vi "ALONE_3AXIS_AMI_DESIM.vi"(6 "Refresco(s)":dbl=1.0, 8 "error in (no error)":errorcluster) -> (0 "Error Out":errorcluster, 7 "Enable":bool=TRUE)   [LabVIEW 2017]
uses:
  AMI MAGNET/Status AMI.ctl
  AMI MAGNET/magneticField.ctl
  ALONE_3AXIS_AMI.ctl
  AMI MAGNET/AMI 430_Hardware_Module.ctl
  AMI MAGNET/commsControl.ctl
  cRIO_ZNB_AMI_GLOBALES.vi
panel:
  in  "Demag X":bool
  out "Remote DEMAG Z":bool
  out "Remote DEMAG X":bool
  out "Remote DEMAG Y":bool
  in  "Demag Y":bool
  in  "Demag Z":bool
  out "String":string="Estado"
  out "Command":T1
  out "Remote RAMP Z":bool
  out "Remote SET X":bool
  out "Remote SET Y":bool
  out "Remote RAMP X":bool
  out "Remote RAMP Y":bool
  out "Remote SET Z":bool
  in  "rampingMode X":u16(ring)=1 items=["RAMP", "PAUSE", "MANUAL UP", "MANUAL DOWN", "ZERO"]
  in  "rampingMode Y":u16(ring)=1 items=["RAMP", "PAUSE", "MANUAL UP", "MANUAL DOWN", "ZERO"]
  in  "rampingMode Z":u16(ring)=1 items=["RAMP", "PAUSE", "MANUAL UP", "MANUAL DOWN", "ZERO"]
  in  "RAMP Z":bool
  in  "SET X":bool
  out "X ramping":bool caption="Stable"
  out "X state":T2=1 items=["Unknown", "RAMPING to target field/current", "HOLDING at the target field/current", "PAUSED", "Ramping in MANUAL UP mode", "Ramping in MANUAL DOWN mode", "ZEROING CURRENT (in progress)", "Quench detected", "At ZERO current", "Heating persistent switch", "Cooling persistent switch", "External Rampdown active"]
  in  "Target X(T)":dbl min=-0.5 max=0.5 step=0.001 format="%.3f"
  in  "Rate X(T/min)":dbl=0.1 min=0.0 max=0.1 step=0.001 format="%.3f"
  out "X field (T)":dbl format="%.3f"
  in  "SET Y":bool
  out "Y ramping":bool caption="Stable"
  out "Y state":T2=1 items=["Unknown", "RAMPING to target field/current", "HOLDING at the target field/current", "PAUSED", "Ramping in MANUAL UP mode", "Ramping in MANUAL DOWN mode", "ZEROING CURRENT (in progress)", "Quench detected", "At ZERO current", "Heating persistent switch", "Cooling persistent switch", "External Rampdown active"]
  in  "Target Y(T)":dbl min=-0.5 max=0.5 step=0.001 format="%.3f"
  in  "Rate Y(T/min)":dbl=0.1 min=0.0 max=0.1 step=0.001 format="%.3f"
  out "Y field (T)":dbl format="%.3f"
  in  "RAMP X":bool
  in  "RAMP Y":bool
  in  "Settings Z":T3={"magneticFieldUnits"=1, "rampRateUnits"=1, "rampRate"=0.0, "targetField"=0.0, "rampingMode"=1} {"rampingMode" items=["RAMP", "PAUSE", "MANUAL UP", "MANUAL DOWN", "ZERO"]; "targetField" format="%.3f"; "rampRate" format="%.3f"; "rampRateUnits" items=["Per SECOND", "Per MINUTE"]; "magneticFieldUnits" items=["KGauss", "Tesla"]}
  in  "Settings Y":T3={"magneticFieldUnits"=1, "rampRateUnits"=1, "rampRate"=0.0, "targetField"=0.0, "rampingMode"=1} {"rampingMode" items=["RAMP", "PAUSE", "MANUAL UP", "MANUAL DOWN", "ZERO"]; "targetField" format="%.3f"; "rampRate" format="%.3f"; "rampRateUnits" items=["Per SECOND", "Per MINUTE"]; "magneticFieldUnits" items=["KGauss", "Tesla"]}
  in  "Settings X":T3={"magneticFieldUnits"=1, "rampRateUnits"=1, "rampRate"=0.0, "targetField"=0.0, "rampingMode"=1} {"rampingMode" items=["RAMP", "PAUSE", "MANUAL UP", "MANUAL DOWN", "ZERO"]; "targetField" format="%.3f"; "rampRate" format="%.3f"; "rampRateUnits" items=["Per SECOND", "Per MINUTE"]; "magneticFieldUnits" items=["KGauss", "Tesla"]}
  out "Waveform Chart":T4(graph)
  in  "SET Z":bool
  out "Z ramping":bool caption="Stable"
  out "Z state":T2=1 items=["Unknown", "RAMPING to target field/current", "HOLDING at the target field/current", "PAUSED", "Ramping in MANUAL UP mode", "Ramping in MANUAL DOWN mode", "ZEROING CURRENT (in progress)", "Quench detected", "At ZERO current", "Heating persistent switch", "Cooling persistent switch", "External Rampdown active"]
  out "Ciclo":i32
  in  "Target Z(T)":dbl min=-2.0 max=2.0 step=0.001 format="%.3f"
  in  "Rate Z(T/min)":dbl=0.1 min=0.0 max=0.1 step=0.001 format="%.3f"
  out "Z field (T)":dbl format="%.3f"
  out "ERROR":bool
  out "Date":string caption="asd"
  out "Time":string caption="asd"
  in  "Refresh":bool
  in  "stop":bool
  # "Z axis"
  # "Y axis"
  # "X axis"
  # "STATUS"
  # "STATUS"
  # "STATUS"
  # "SETTINGS"
  # "SETTINGS"
  # "SETTINGS"
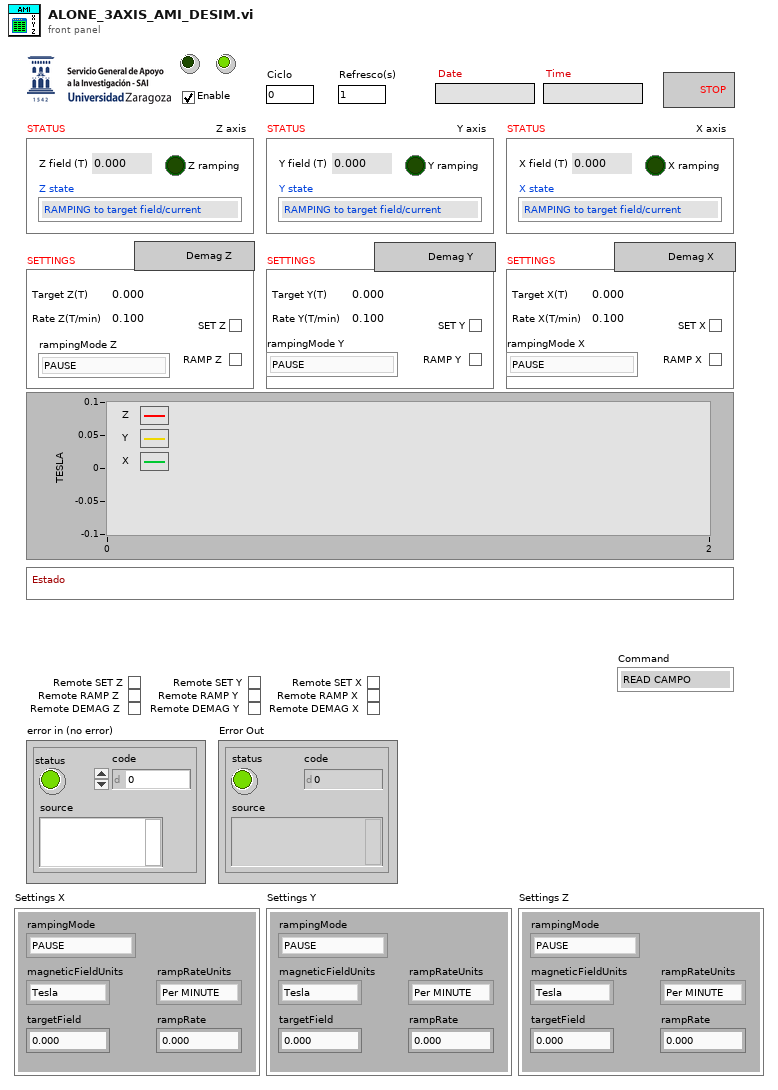
[diagram p1: front panel]
types:
  T1 = typedef "ALONE_3AXIS_AMI.ctl" = enum16{"READ CAMPO", "SET X", "SET Y", "SET Z", "RAMP X", "RAMP Y", "RAMP Z", "DESIMANAR X", "DESIMANAR Y", "DESIMANAR Z", "DESIMANAR X_RUN", "DESIMANAR Y_RUN", "DESIMANAR Z_RUN"}
  T2 = typedef "Status AMI.ctl" = u16
  T3 = typedef "magneticField.ctl" = cluster{"magneticFieldUnits":u16, "rampRateUnits":u16, "rampRate":dbl, "targetField":dbl, "rampingMode":u16}
  T4 = cluster{"magneticField":dbl, "magneticField":dbl, "magneticField":dbl}
  T5 = typedef "AMI 430_Hardware_Module.ctl" = enum16{"INICIALIZAR", "SET UNIDADES CAMPO", "SET UNIDADES RAMPA", "SET CAMPO", "SET  RAMPA", "SET RAMPING MODE", "READ CAMPO", "STATUS", "SHUTDOWN"}
  T6 = typedef "commsControl.ctl" = cluster{"connection ID":refnum<k5>, "IP":string, "Active Comm Interface":u16, "Serial Port":refnum<visa-resource-name>, "Programmer Type":u16, "connection ID":refnum<k5>, "output cluster":cluster{"GPIB address":i16, "GPIB bus":i16}}
  T7 = cluster{"Z field (T)":dbl, "Y field (T)":dbl, "magneticField":dbl}
  T8 = cluster{"Z field (T)":dbl, "magneticField":dbl, "X field (T)":dbl}
  T9 = cluster{"magneticField":dbl, "Y field (T)":dbl, "X field (T)":dbl}
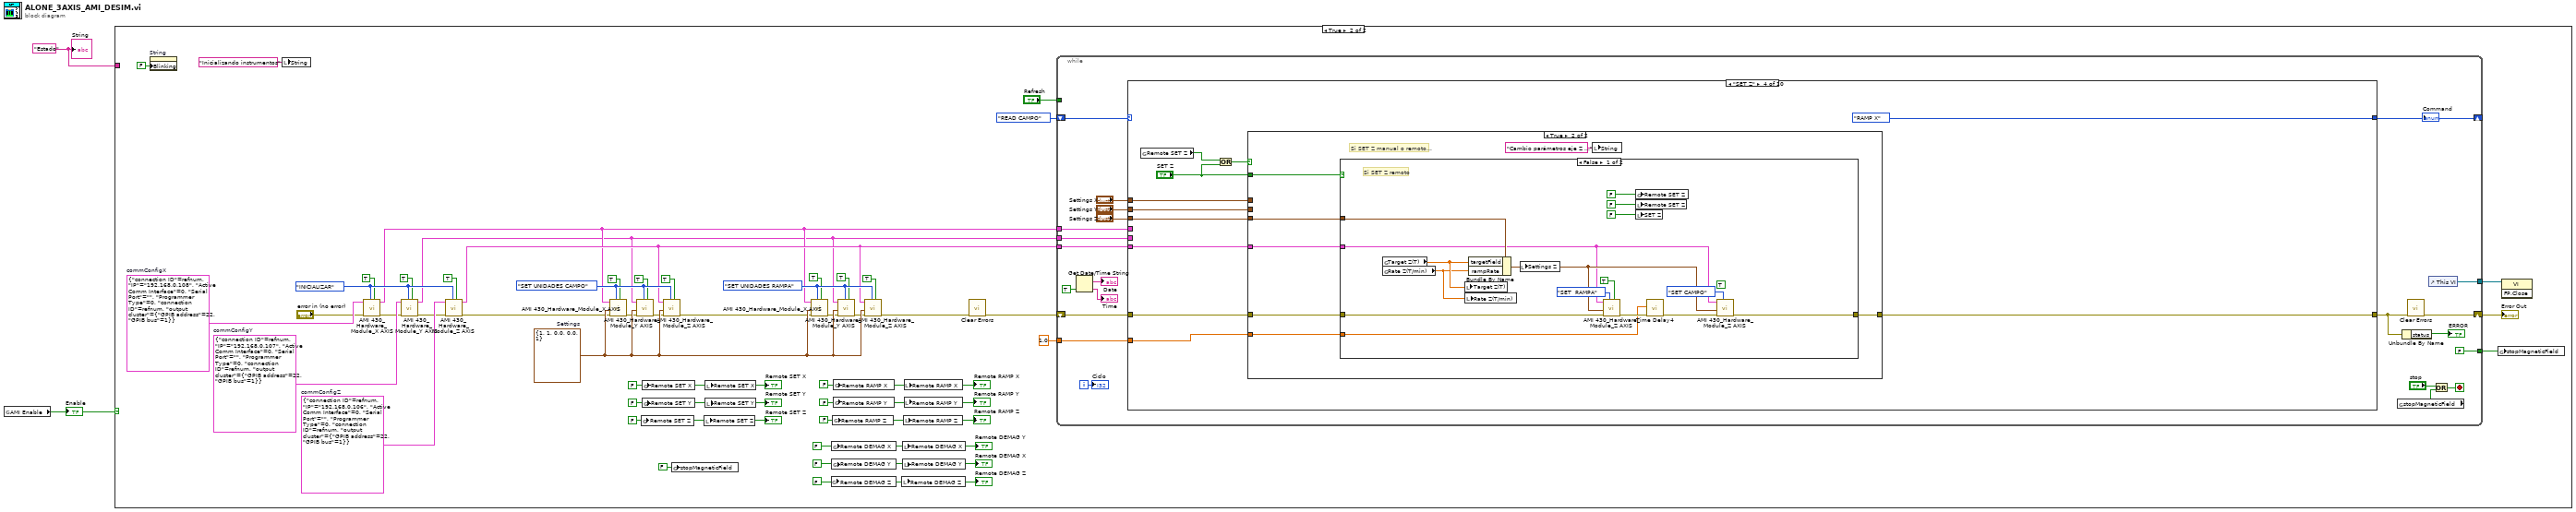
[diagram p0: block diagram]
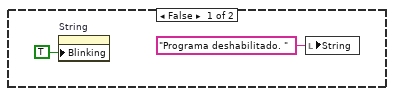
[diagram p2: hidden frame]
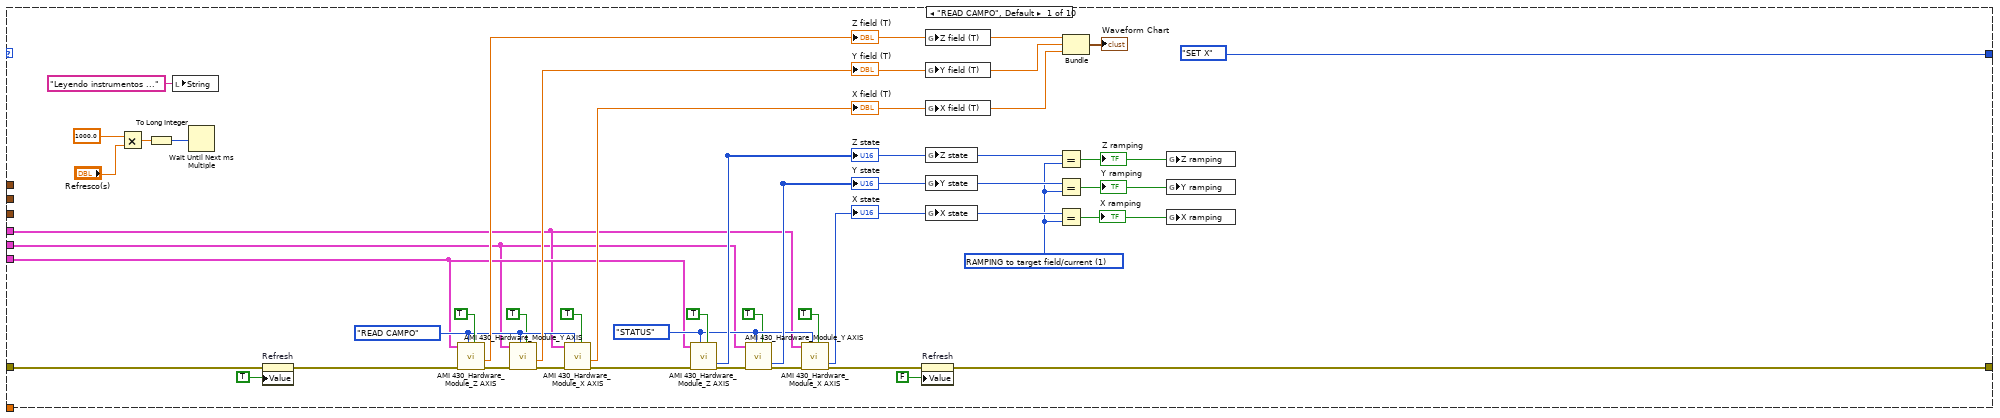
[diagram p3: hidden frame]
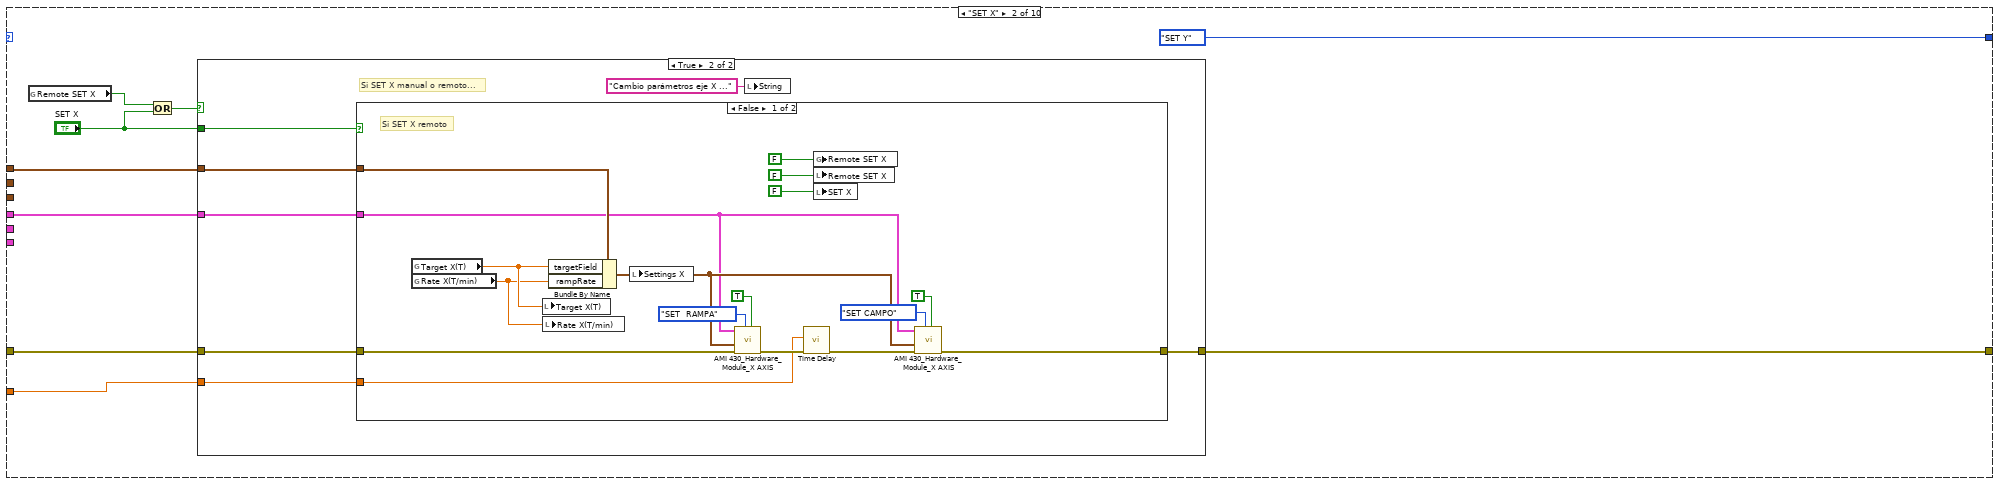
[diagram p4: hidden frame]
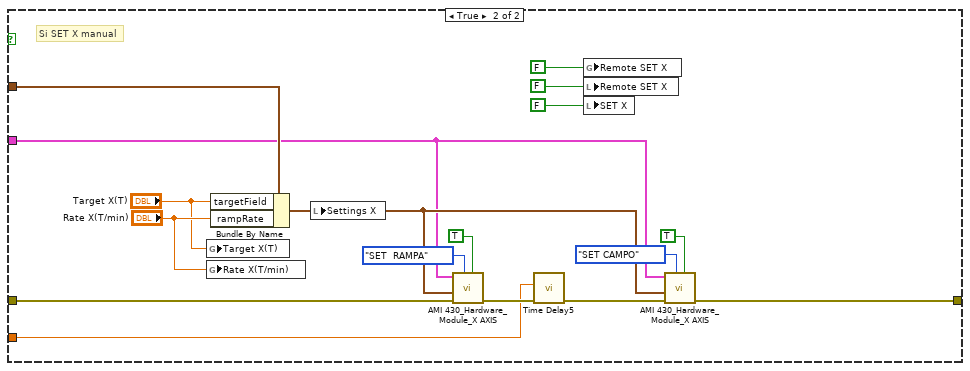
[diagram p6: hidden frame]
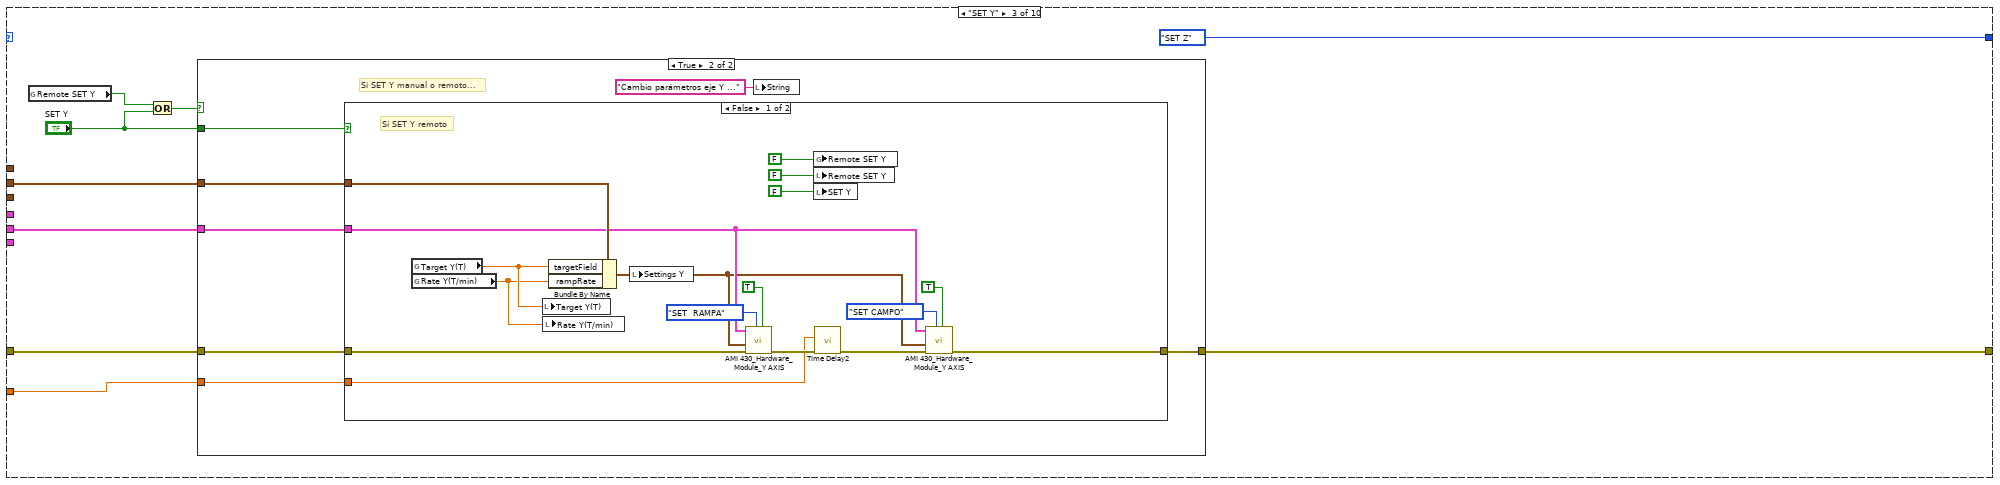
[diagram p7: hidden frame]
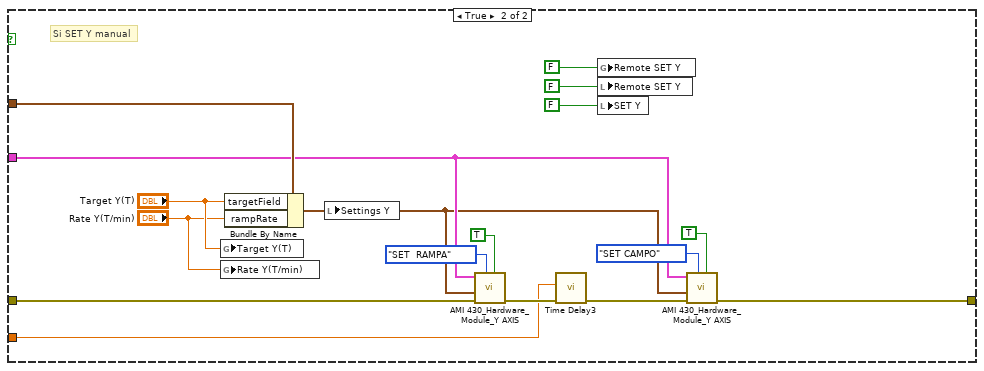
[diagram p9: hidden frame]
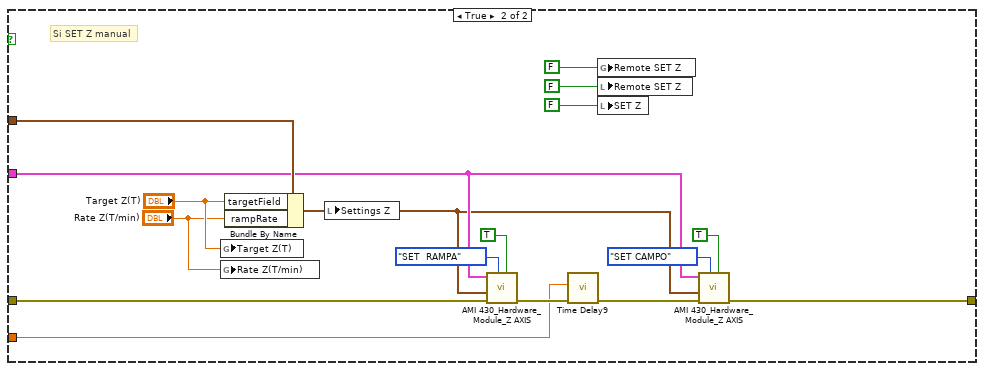
[diagram p11: hidden frame]
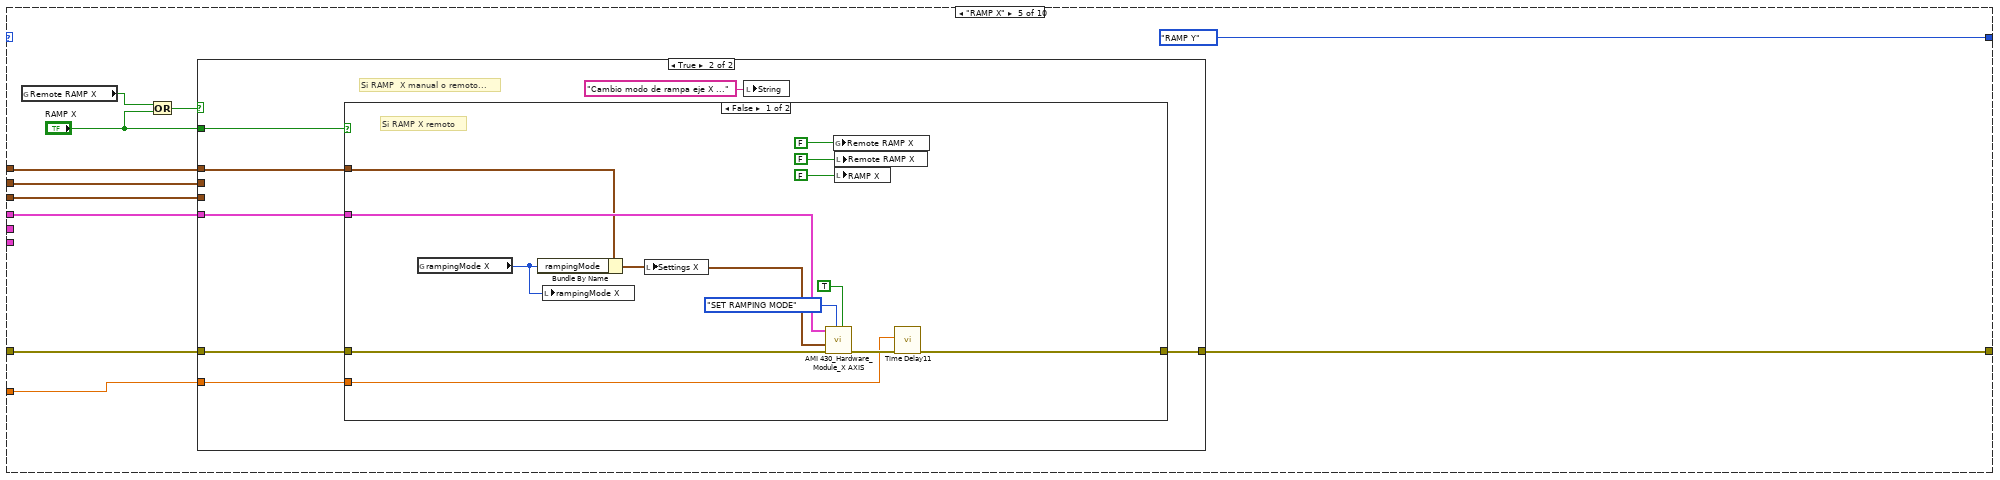
[diagram p12: hidden frame]
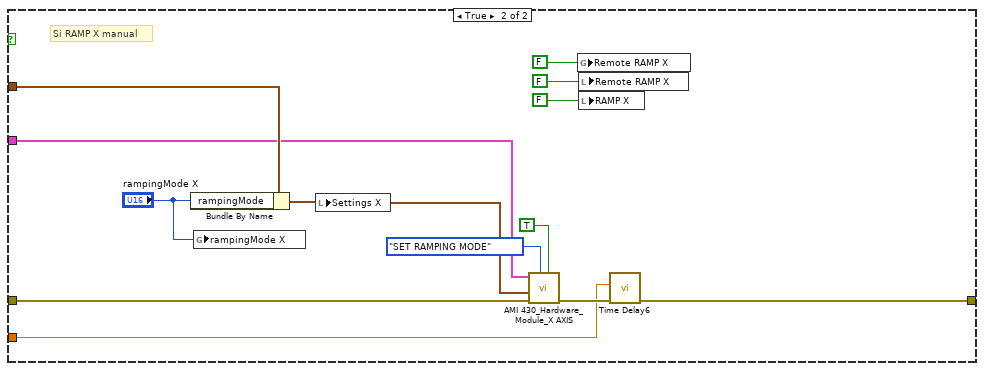
[diagram p14: hidden frame]
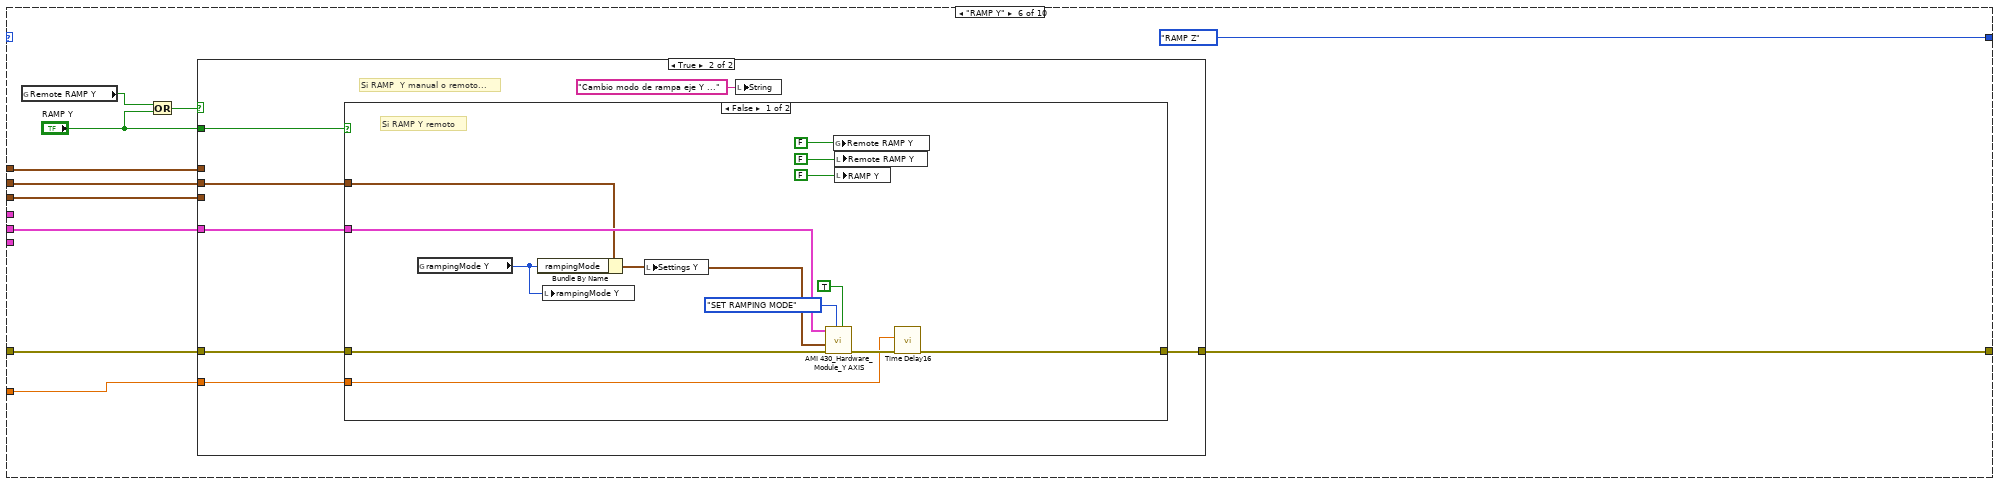
[diagram p15: hidden frame]
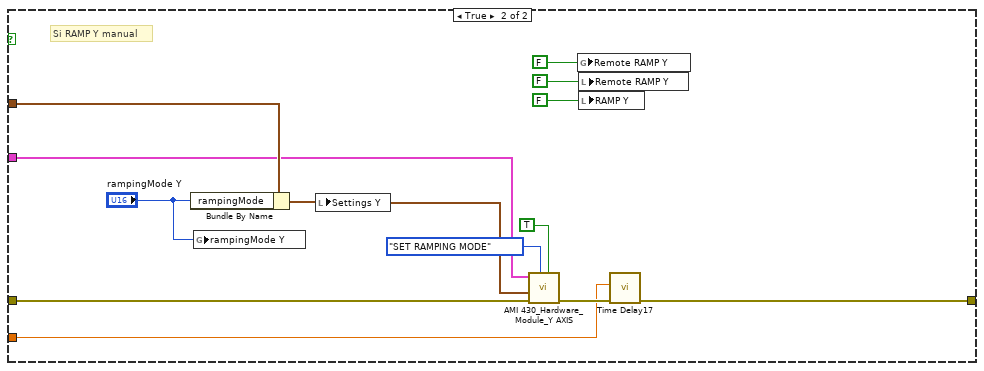
[diagram p17: hidden frame]
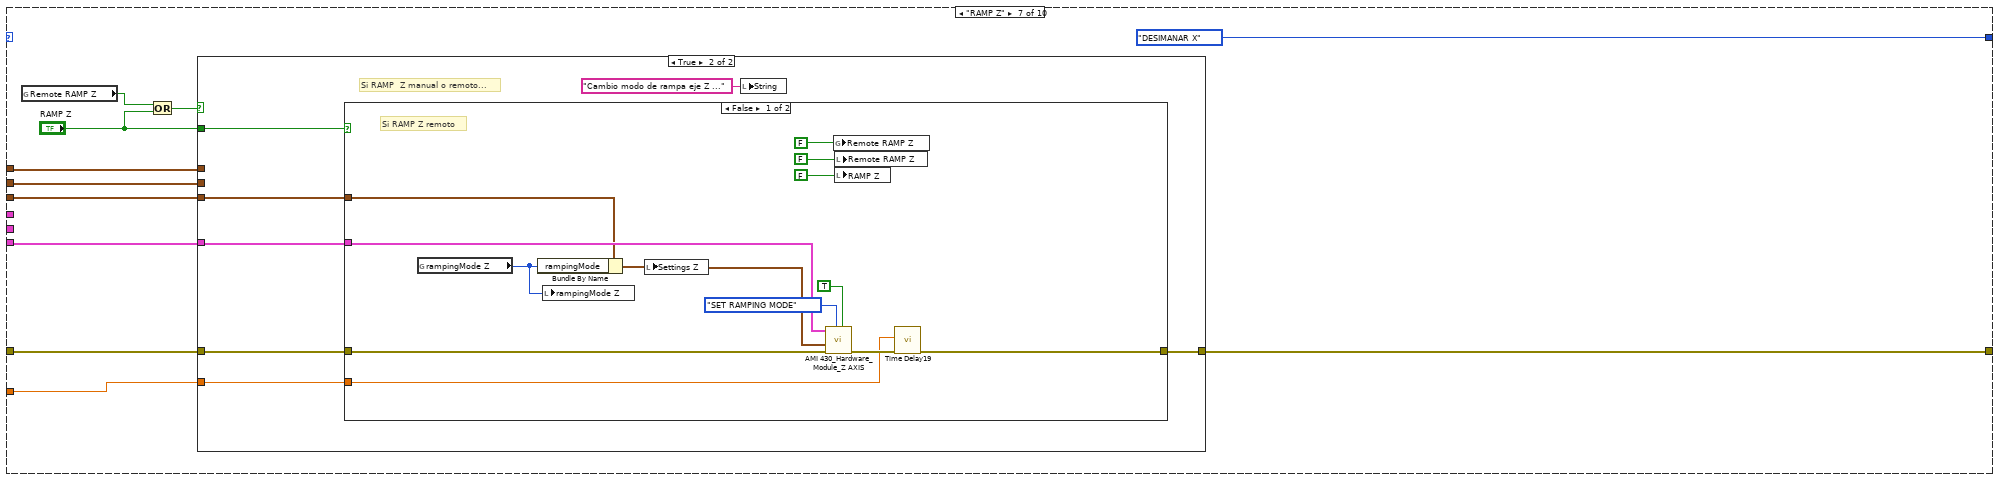
[diagram p18: hidden frame]
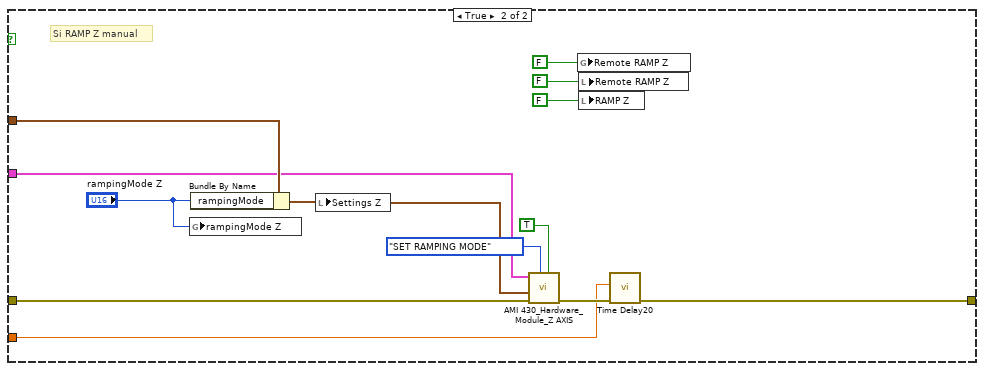
[diagram p20: hidden frame]
diagram:
  w1 = "Estado" ("String")
  n1 = global read "cRIO_ZNB_AMI_GLOBALES.vi" "AMI Enable"() -> (w2:bool)
  "Enable" <- w2
  n2 = case shown="True" w2 {
    tunnel: w1 -> [_ _]
    frame False {
      n3 = property on="String" class="Str"("Blinking"=TRUE) -> ()  [unwired: 2 in, 2 out]
      n4 = local write "String"("Programa deshabilitado. " ("String")) -> ()
    }
    frame True {
      w5 = FALSE ("Remote RAMP Z")
      w6 = FALSE ("Remote RAMP Y")
      w7 = FALSE ("Remote RAMP X")
      w12 = FALSE ("Remote SET Z")
      w11 = FALSE ("Remote SET Y")
      w13 = FALSE ("Remote SET X")
      w16 = FALSE ("Remote RAMP Z")
      w15 = FALSE ("Remote RAMP Y")
      w14 = FALSE ("Remote RAMP X")
      w45 = T3 {"magneticFieldUnits"=1, "rampRateUnits"=1, "rampRate"=0.0, "targetField"=0.0, "rampingMode"=1}  # Settings
      w41 = AMI_430_Hardware_Module."SET UNIDADES RAMPA" ("Command")
      w40 = AMI_430_Hardware_Module."SET UNIDADES CAMPO" ("Command")
      w48 = T6 {"connection ID"=refnum, "IP"="192.168.0.106", "Active Comm Interface"=0, "Serial Port"="", "Programmer Type"=0, "connection ID"=refnum, "output cluster"={"GPIB address"=22, "GPIB bus"=1}}  # commConfigZ
      w47 = T6 {"connection ID"=refnum, "IP"="192.168.0.107", "Active Comm Interface"=0, "Serial Port"="", "Programmer Type"=0, "connection ID"=refnum, "output cluster"={"GPIB address"=22, "GPIB bus"=1}}  # commConfigY
      w46 = T6 {"connection ID"=refnum, "IP"="192.168.0.108", "Active Comm Interface"=0, "Serial Port"="", "Programmer Type"=0, "connection ID"=refnum, "output cluster"={"GPIB address"=22, "GPIB bus"=1}}  # commConfigX
      w49 = AMI_430_Hardware_Module."INICIALIZAR" ("Command")
      n5 = property on="String" class="Str"("Blinking"=FALSE) -> ()  [unwired: 2 in, 2 out]
      n6 = local write "String"("Inicializando instrumentos" ("String")) -> ()
      n7 = call "AMI 430_Hardware_Module_X AXIS.vi"("Enable"=TRUE, "Command"=w49, "error in (no error)"="error in (no error)", "Comm Config In"=w46) -> ("error out"=w36:errorcluster, "Comm Config Out"=w20:T6)  [unwired: 3 in, 3 out]
      n8 = call "AMI 430_Hardware_Module_Y AXIS.vi"("Enable"=TRUE, "Command"=w49, "error in (no error)"=w36, "Comm Config In"=w47) -> ("error out"=w35:errorcluster, "Comm Config Out"=w19:T6)  [unwired: 3 in, 3 out]
      n9 = call "AMI 430_Hardware_Module_Z AXIS.vi"("Enable"=TRUE, "Command"=w49, "error in (no error)"=w35, "Comm Config In"=w48) -> ("error out"=w39:errorcluster, "Comm Config Out"=w21:T6)  [unwired: 3 in, 3 out]
      n10 = call "AMI 430_Hardware_Module_X AXIS.vi"("Enable"=TRUE, "Command"=w40, "error in (no error)"=w39, "Settings"=w45, "Comm Config In"=w20) -> ("error out"=w37:errorcluster)  [unwired: 2 in, 4 out]
      n11 = call "AMI 430_Hardware_Module_Y AXIS.vi"("Enable"=TRUE, "Command"=w40, "error in (no error)"=w37, "Settings"=w45, "Comm Config In"=w19) -> ("error out"=w38:errorcluster)  [unwired: 2 in, 4 out]
      n12 = global write "cRIO_ZNB_AMI_GLOBALES.vi" "Remote SET Z"(w12) -> ()
      n13 = global write "cRIO_ZNB_AMI_GLOBALES.vi" "Remote SET X"(w13) -> ()
      n14 = global write "cRIO_ZNB_AMI_GLOBALES.vi" "Remote SET Y"(w11) -> ()
      n15 = call "AMI 430_Hardware_Module_Z AXIS.vi"("Enable"=TRUE, "Command"=w40, "error in (no error)"=w38, "Settings"=w45, "Comm Config In"=w21) -> ("error out"=w44:errorcluster)  [unwired: 2 in, 4 out]
      n16 = global write "cRIO_ZNB_AMI_GLOBALES.vi" "stopMagneticField"(FALSE ("stopMagneticField")) -> ()
      n17 = local write "Remote SET Z"(w12) -> ()
      n18 = local write "Remote SET X"(w13) -> ()
      n19 = local write "Remote SET Y"(w11) -> ()
      n20 = call "AMI 430_Hardware_Module_X AXIS.vi"("Enable"=TRUE, "Command"=w41, "error in (no error)"=w44, "Settings"=w45, "Comm Config In"=w20) -> ("error out"=w42:errorcluster)  [unwired: 2 in, 4 out]
      n21 = global write "cRIO_ZNB_AMI_GLOBALES.vi" "Remote DEMAG Z"(w5) -> ()
      n22 = global write "cRIO_ZNB_AMI_GLOBALES.vi" "Remote DEMAG X"(w7) -> ()
      n23 = global write "cRIO_ZNB_AMI_GLOBALES.vi" "Remote DEMAG Y"(w6) -> ()
      n24 = global write "cRIO_ZNB_AMI_GLOBALES.vi" "Remote RAMP Z"(w16) -> ()
      n25 = global write "cRIO_ZNB_AMI_GLOBALES.vi" "Remote RAMP X"(w14) -> ()
      n26 = global write "cRIO_ZNB_AMI_GLOBALES.vi" "Remote RAMP Y"(w15) -> ()
      n27 = call "AMI 430_Hardware_Module_Y AXIS.vi"("Enable"=TRUE, "Command"=w41, "error in (no error)"=w42, "Settings"=w45, "Comm Config In"=w19) -> ("error out"=w43:errorcluster)  [unwired: 2 in, 4 out]
      n28 = call "AMI 430_Hardware_Module_Z AXIS.vi"("Enable"=TRUE, "Command"=w41, "error in (no error)"=w43, "Settings"=w45, "Comm Config In"=w21) -> ("error out"=w34:errorcluster)  [unwired: 2 in, 4 out]
      n29 = local write "Remote DEMAG Z"(w5) -> ()
      n30 = local write "Remote DEMAG X"(w7) -> ()
      n31 = local write "Remote DEMAG Y"(w6) -> ()
      n32 = local write "Remote RAMP Z"(w16) -> ()
      n33 = local write "Remote RAMP X"(w14) -> ()
      n34 = local write "Remote RAMP Y"(w15) -> ()
      n35 = call <vilib>:"Clear Errors.vi"("error in (no error)"=w34) -> ("error out"=w18:errorcluster)  [unwired: 5 in, 1 out]
      n36 = while {
        shift-right: [w65] -> w50
        shift-left: w18 -> [w58]
        tunnel: [FALSE ("stop")] -> w51
        tunnel: [w68] -> w52
        tunnel: "Refresh" -> [_]
        tunnel: w19 -> [w59]
        tunnel: w21 -> [w60]
        tunnel: w20 -> [w61]
        shift-right: [w54] -> _
        shift-left: ALONE_3AXIS_AMI."READ CAMPO" ("Command") -> [w63]
        tunnel: 1.0 ("Delay Time (s)") -> [w53]
        i -> [w64]
        stop <- w72 stop-if-true
        n37 = Get Date/Time String(want seconds? (F)=TRUE) -> (date string=→"Date":string, time string=→"Time":string)  [unwired: 2 in]
        n38 = case shown="\"SET Z\"" w63 {
          tunnel: w58 -> [w78 w121 w173 w225 w277 w322 w367 w412 w496 w581]
          tunnel: w61 -> [w88 w117 _ _ w268 _ _ w404 _ _]
          tunnel: w59 -> [w87 _ w165 _ _ w314 _ _ w487 _]
          tunnel: w60 -> [w89 _ _ w216 _ _ w358 _ _ w572]
          tunnel: [w75 w120 w172 w224 w276 w321 w366 w411 w495 w580] -> w62
          tunnel: "Settings Y" -> [_ _ w166 w217 w270 w315 w360 w405 w489 w574]
          tunnel: "Settings Z" -> [_ _ _ w218 w271 w316 w361 w406 w490 w575]
          tunnel: "Settings X" -> [_ w122 _ w226 w278 w323 w368 w413 w497 w582]
          tunnel: [ALONE_3AXIS_AMI."SET X" ("Command") ALONE_3AXIS_AMI."SET Y" ("Command") ALONE_3AXIS_AMI."SET Z" ("Command") ALONE_3AXIS_AMI."RAMP X" ("Command") ALONE_3AXIS_AMI."RAMP Y" ("Command") ALONE_3AXIS_AMI."RAMP Z" ("Command") ALONE_3AXIS_AMI."DESIMANAR X" ("Command") ALONE_3AXIS_AMI."DESIMANAR Y" ("Command") ALONE_3AXIS_AMI."DESIMANAR Z" ("Command") ALONE_3AXIS_AMI."READ CAMPO" ("Command")] -> w54
          tunnel: w53 -> [_ w118 w170 w222 w274 w319 w364 w409 w493 w578]
          frame "READ CAMPO", Default {
            w98 = T2 1 items=["Unknown", "RAMPING to target field/current", "HOLDING at the target field/current", "PAUSED", "Ramping in MANUAL UP mode", "Ramping in MANUAL DOWN mode", "ZEROING CURRENT (in progress)", "Quench detected", "At ZERO current", "Heating persistent switch", "Cooling persistent switch", "External Rampdown active"] ("y")
            w96 = AMI_430_Hardware_Module."STATUS" ("Command")
            w92 = AMI_430_Hardware_Module."READ CAMPO" ("Command")
            n39 = Multiply(x=1000.0, y="Refresco(s)") -> (x*y=w83:dbl)
            n40 = To Long Integer(number=w83) -> (32bit integer=w81:i32)
            n41 = local write "String"("Leyendo instrumentos ..." ("String")) -> ()
            n42 = Wait Until Next ms Multiple(millisecond multiple=w81) -> ()  [unwired: 1 out]
            n43 = property on="Refresh" class="Bool (strict)"(error in=w78, "Value"=TRUE ("Refresh")) -> (error out=w77:errorcluster)  [unwired: 1 in, 1 out]
            n44 = call "AMI 430_Hardware_Module_Z AXIS.vi"("Enable"=TRUE, "Command"=w92, "error in (no error)"=w77, "Comm Config In"=w89) -> ("error out"=w100:errorcluster, "magneticField"=w110:dbl)  [unwired: 3 in, 3 out]
            "Z field (T)" <- w110
            n45 = call "AMI 430_Hardware_Module_Y AXIS.vi"("Enable"=TRUE, "Command"=w92, "error in (no error)"=w100, "Comm Config In"=w87) -> ("error out"=w99:errorcluster, "magneticField"=w109:dbl)  [unwired: 3 in, 3 out]
            "Y field (T)" <- w109
            n46 = call "AMI 430_Hardware_Module_X AXIS.vi"("Enable"=TRUE, "Command"=w92, "error in (no error)"=w99, "Comm Config In"=w88) -> ("error out"=w101:errorcluster, "magneticField"=w108:dbl)  [unwired: 3 in, 3 out]
            "X field (T)" <- w108
            n47 = call "AMI 430_Hardware_Module_Z AXIS.vi"("Enable"=TRUE, "Command"=w96, "error in (no error)"=w101, "Comm Config In"=w89) -> ("error out"=w103:errorcluster, "state"=w111:T2)  [unwired: 3 in, 3 out]
            "Z state" <- w111
            n48 = call "AMI 430_Hardware_Module_Y AXIS.vi"("Enable"=TRUE, "Command"=w96, "error in (no error)"=w103, "Comm Config In"=w87) -> ("error out"=w102:errorcluster, "state"=w112:T2)  [unwired: 3 in, 3 out]
            "Y state" <- w112
            n49 = call "AMI 430_Hardware_Module_X AXIS.vi"("Enable"=TRUE, "Command"=w96, "error in (no error)"=w102, "Comm Config In"=w88) -> ("error out"=w76:errorcluster, "state"=w113:T2)  [unwired: 3 in, 3 out]
            "X state" <- w113
            n50 = property on="Refresh" class="Bool (strict)"(error in=w76, "Value"=FALSE ("Refresh")) -> (error out=w75:errorcluster)  [unwired: 1 in, 1 out]
            n51 = global write "cRIO_ZNB_AMI_GLOBALES.vi" "Z field (T)"(w110) -> ()
            n52 = global write "cRIO_ZNB_AMI_GLOBALES.vi" "Y field (T)"(w109) -> ()
            n53 = global write "cRIO_ZNB_AMI_GLOBALES.vi" "X field (T)"(w108) -> ()
            n54 = global write "cRIO_ZNB_AMI_GLOBALES.vi" "Z state"(w111) -> ()
            n55 = global write "cRIO_ZNB_AMI_GLOBALES.vi" "Y state"(w112) -> ()
            n56 = global write "cRIO_ZNB_AMI_GLOBALES.vi" "X state"(w113) -> ()
            n57 = Equal?(x=w111, y=w98) -> (x = y?=w105:bool)
            "Z ramping" <- w105
            n58 = Equal?(x=w112, y=w98) -> (x = y?=w107:bool)
            "Y ramping" <- w107
            n59 = Equal?(x=w113, y=w98) -> (x = y?=w106:bool)
            "X ramping" <- w106
            n60 = Bundle("magneticField"=w110, "magneticField"=w109, "magneticField"=w108) -> (→"Waveform Chart":T4)  [unwired: 1 in]
            n61 = global write "cRIO_ZNB_AMI_GLOBALES.vi" "Z ramping"(w105) -> ()
            n62 = global write "cRIO_ZNB_AMI_GLOBALES.vi" "Y ramping"(w107) -> ()
            n63 = global write "cRIO_ZNB_AMI_GLOBALES.vi" "X ramping"(w106) -> ()
          }
          frame "SET X" {
            n64 = global read "cRIO_ZNB_AMI_GLOBALES.vi" "Remote SET X"() -> (w116:bool)
            n65 = Or(x=w116, y="SET X") -> (x .or. y?=w115:bool)
            n66 = case shown="True" w115 {
              tunnel: w122 -> [_ w130]
              tunnel: w121 -> [w123 w129]
              tunnel: [w123 w128] -> w120
              tunnel: w118 -> [_ w127]
              tunnel: w117 -> [_ w126]
              tunnel: "SET X" -> [_ w125]
              frame False {
              }
              frame True {
                # "Si SET X manual o remoto..."
                n67 = case shown="False" w125 {
                  tunnel: w130 -> [w140 w155]
                  tunnel: w129 -> [w139 w154]
                  tunnel: [w138 w153] -> w128
                  tunnel: w127 -> [w137 w152]
                  tunnel: w126 -> [w136 w151]
                  frame False {
                    # "Si SET X remoto"
                    n68 = global read "cRIO_ZNB_AMI_GLOBALES.vi" "Target X(T)"() -> (w135:dbl)
                    n69 = global read "cRIO_ZNB_AMI_GLOBALES.vi" "Rate X(T/min)"() -> (w134:dbl)
                    n70 = local write "Target X(T)"(w135) -> ()
                    n71 = local write "Rate X(T/min)"(w134) -> ()
                    n72 = Bundle By Name(cluster=w140, "targetField"=w135, "rampRate"=w134) -> (w147:T3)
                    n73 = local write "Settings X"(w147) -> ()
                    n74 = call "AMI 430_Hardware_Module_X AXIS.vi"("Enable"=TRUE, "Command"=AMI_430_Hardware_Module."SET  RAMPA", "error in (no error)"=w139, "Settings"=w147, "Comm Config In"=w136) -> ("error out"=w145:errorcluster)  [unwired: 2 in, 4 out]
                    n75 = call "Time Delay"("error in (no error)"=w145, "Delay Time (s)"=w137) -> ("error out"=w146:errorcluster)  [unwired: 9 in]
                    n76 = global write "cRIO_ZNB_AMI_GLOBALES.vi" "Remote SET X"(FALSE ("Remote SET X")) -> ()
                    n77 = local write "Remote SET X"(FALSE ("Remote SET X")) -> ()
                    n78 = local write "SET X"(FALSE ("Remote SET X")) -> ()
                    n79 = call "AMI 430_Hardware_Module_X AXIS.vi"("Enable"=TRUE, "Command"=AMI_430_Hardware_Module."SET CAMPO", "error in (no error)"=w146, "Settings"=w147, "Comm Config In"=w136) -> ("error out"=w138:errorcluster)  [unwired: 2 in, 4 out]
                  }
                  frame True {
                    # "Si SET X manual"
                    n80 = global write "cRIO_ZNB_AMI_GLOBALES.vi" "Target X(T)"("Target X(T)") -> ()
                    n81 = global write "cRIO_ZNB_AMI_GLOBALES.vi" "Rate X(T/min)"("Rate X(T/min)") -> ()
                    n82 = Bundle By Name(cluster=w155, "targetField"="Target X(T)", "rampRate"="Rate X(T/min)") -> (w162:T3)
                    n83 = local write "Settings X"(w162) -> ()
                    n84 = call "AMI 430_Hardware_Module_X AXIS.vi"("Enable"=TRUE, "Command"=AMI_430_Hardware_Module."SET  RAMPA", "error in (no error)"=w154, "Settings"=w162, "Comm Config In"=w151) -> ("error out"=w160:errorcluster)  [unwired: 2 in, 4 out]
                    n85 = call "Time Delay5"("error in (no error)"=w160, "Delay Time (s)"=w152) -> ("error out"=w161:errorcluster)  [unwired: 9 in]
                    n86 = global write "cRIO_ZNB_AMI_GLOBALES.vi" "Remote SET X"(FALSE ("Remote SET X")) -> ()
                    n87 = local write "Remote SET X"(FALSE ("Remote SET X")) -> ()
                    n88 = local write "SET X"(FALSE ("Remote SET X")) -> ()
                    n89 = call "AMI 430_Hardware_Module_X AXIS.vi"("Enable"=TRUE, "Command"=AMI_430_Hardware_Module."SET CAMPO", "error in (no error)"=w161, "Settings"=w162, "Comm Config In"=w151) -> ("error out"=w153:errorcluster)  [unwired: 2 in, 4 out]
                  }
                }
                n90 = local write "String"("Cambio parámetros eje X ..." ("String")) -> ()
              }
            }
          }
          frame "SET Y" {
            n91 = global read "cRIO_ZNB_AMI_GLOBALES.vi" "Remote SET Y"() -> (w169:bool)
            n92 = Or(x=w169, y="SET Y") -> (x .or. y?=w168:bool)
            n93 = case shown="True" w168 {
              tunnel: w166 -> [_ w181]
              tunnel: w173 -> [w174 w180]
              tunnel: [w174 w179] -> w172
              tunnel: w170 -> [_ w178]
              tunnel: w165 -> [_ w177]
              tunnel: "SET Y" -> [_ w176]
              frame False {
              }
              frame True {
                # "Si SET Y manual o remoto..."
                n94 = case shown="False" w176 {
                  tunnel: w181 -> [w198 w215]
                  tunnel: w180 -> [w184 w205]
                  tunnel: [w182 w204] -> w179
                  tunnel: w178 -> [w183 w203]
                  tunnel: w177 -> [w186 w202]
                  frame False {
                    # "Si SET Y remoto"
                    n95 = global read "cRIO_ZNB_AMI_GLOBALES.vi" "Target Y(T)"() -> (w197:dbl)
                    n96 = global read "cRIO_ZNB_AMI_GLOBALES.vi" "Rate Y(T/min)"() -> (w196:dbl)
                    n97 = local write "Target Y(T)"(w197) -> ()
                    n98 = local write "Rate Y(T/min)"(w196) -> ()
                    n99 = Bundle By Name(cluster=w198, "targetField"=w197, "rampRate"=w196) -> (w185:T3)
                    n100 = local write "Settings Y"(w185) -> ()
                    n101 = call "AMI 430_Hardware_Module_Y AXIS.vi"("Enable"=TRUE, "Command"=AMI_430_Hardware_Module."SET  RAMPA", "error in (no error)"=w184, "Settings"=w185, "Comm Config In"=w186) -> ("error out"=w192:errorcluster)  [unwired: 2 in, 4 out]
                    n102 = global write "cRIO_ZNB_AMI_GLOBALES.vi" "Remote SET Y"(FALSE ("Remote SET X")) -> ()
                    n103 = local write "Remote SET Y"(FALSE ("Remote SET X")) -> ()
                    n104 = local write "SET Y"(FALSE ("Remote SET X")) -> ()
                    n105 = call "Time Delay2"("error in (no error)"=w192, "Delay Time (s)"=w183) -> ("error out"=w190:errorcluster)  [unwired: 9 in]
                    n106 = call "AMI 430_Hardware_Module_Y AXIS.vi"("Enable"=TRUE, "Command"=AMI_430_Hardware_Module."SET CAMPO", "error in (no error)"=w190, "Settings"=w185, "Comm Config In"=w186) -> ("error out"=w182:errorcluster)  [unwired: 2 in, 4 out]
                  }
                  frame True {
                    # "Si SET Y manual"
                    n107 = global write "cRIO_ZNB_AMI_GLOBALES.vi" "Target Y(T)"("Target Y(T)") -> ()
                    n108 = global write "cRIO_ZNB_AMI_GLOBALES.vi" "Rate Y(T/min)"("Rate Y(T/min)") -> ()
                    n109 = Bundle By Name(cluster=w215, "targetField"="Target Y(T)", "rampRate"="Rate Y(T/min)") -> (w201:T3)
                    n110 = local write "Settings Y"(w201) -> ()
                    n111 = call "AMI 430_Hardware_Module_Y AXIS.vi"("Enable"=TRUE, "Command"=AMI_430_Hardware_Module."SET  RAMPA", "error in (no error)"=w205, "Settings"=w201, "Comm Config In"=w202) -> ("error out"=w211:errorcluster)  [unwired: 2 in, 4 out]
                    n112 = call "Time Delay3"("error in (no error)"=w211, "Delay Time (s)"=w203) -> ("error out"=w209:errorcluster)  [unwired: 9 in]
                    n113 = global write "cRIO_ZNB_AMI_GLOBALES.vi" "Remote SET Y"(FALSE ("Remote SET X")) -> ()
                    n114 = local write "Remote SET Y"(FALSE ("Remote SET X")) -> ()
                    n115 = local write "SET Y"(FALSE ("Remote SET X")) -> ()
                    n116 = call "AMI 430_Hardware_Module_Y AXIS.vi"("Enable"=TRUE, "Command"=AMI_430_Hardware_Module."SET CAMPO", "error in (no error)"=w209, "Settings"=w201, "Comm Config In"=w202) -> ("error out"=w204:errorcluster)  [unwired: 2 in, 4 out]
                  }
                }
                n117 = local write "String"("Cambio parámetros eje Y ..." ("String")) -> ()
              }
            }
          }
          frame "SET Z" {
            n118 = global read "cRIO_ZNB_AMI_GLOBALES.vi" "Remote SET Z"() -> (w221:bool)
            n119 = Or(x=w221, y="SET Z") -> (x .or. y?=w220:bool)
            n120 = case shown="True" w220 {
              tunnel: w226 -> [_ _]
              tunnel: w225 -> [w227 w234]
              tunnel: [w227 w233] -> w224
              tunnel: w222 -> [_ w232]
              tunnel: w216 -> [_ w231]
              tunnel: "SET Z" -> [_ w230]
              tunnel: w218 -> [_ w229]
              tunnel: w217 -> [_ _]
              frame False {
              }
              frame True {
                # "Si SET Z manual o remoto..."
                n121 = case shown="False" w230 {
                  tunnel: w229 -> [w250 w267]
                  tunnel: w234 -> [w238 w257]
                  tunnel: [w237 w256] -> w233
                  tunnel: w232 -> [w239 w253]
                  tunnel: w231 -> [w235 w255]
                  frame False {
                    (unwired) TRUE ("Enable")
                    # "Si SET Z remoto"
                    n122 = global read "cRIO_ZNB_AMI_GLOBALES.vi" "Target Z(T)"() -> (w249:dbl)
                    n123 = global read "cRIO_ZNB_AMI_GLOBALES.vi" "Rate Z(T/min)"() -> (w248:dbl)
                    n124 = local write "Target Z(T)"(w249) -> ()
                    n125 = local write "Rate Z(T/min)"(w248) -> ()
                    n126 = Bundle By Name(cluster=w250, "targetField"=w249, "rampRate"=w248) -> (w236:T3)
                    n127 = local write "Settings Z"(w236) -> ()
                    n128 = call "AMI 430_Hardware_Module_Z AXIS.vi"("Enable"=TRUE, "Command"=AMI_430_Hardware_Module."SET  RAMPA", "error in (no error)"=w238, "Settings"=w236, "Comm Config In"=w235) -> ("error out"=w241:errorcluster)  [unwired: 2 in, 4 out]
                    n129 = global write "cRIO_ZNB_AMI_GLOBALES.vi" "Remote SET Z"(FALSE ("Remote SET X")) -> ()
                    n130 = local write "Remote SET Z"(FALSE ("Remote SET X")) -> ()
                    n131 = local write "SET Z"(FALSE ("Remote SET X")) -> ()
                    n132 = call "Time Delay4"("error in (no error)"=w241, "Delay Time (s)"=w239) -> ("error out"=w240:errorcluster)  [unwired: 9 in]
                    n133 = call "AMI 430_Hardware_Module_Z AXIS.vi"("Command"=AMI_430_Hardware_Module."SET CAMPO", "error in (no error)"=w240, "Settings"=w236, "Comm Config In"=w235) -> ("error out"=w237:errorcluster)  [unwired: 3 in, 4 out]
                  }
                  frame True {
                    # "Si SET Z manual"
                    n134 = global write "cRIO_ZNB_AMI_GLOBALES.vi" "Target Z(T)"("Target Z(T)") -> ()
                    n135 = global write "cRIO_ZNB_AMI_GLOBALES.vi" "Rate Z(T/min)"("Rate Z(T/min)") -> ()
                    n136 = Bundle By Name(cluster=w267, "targetField"="Target Z(T)", "rampRate"="Rate Z(T/min)") -> (w254:T3)
                    n137 = local write "Settings Z"(w254) -> ()
                    n138 = call "AMI 430_Hardware_Module_Z AXIS.vi"("Enable"=TRUE, "Command"=AMI_430_Hardware_Module."SET  RAMPA", "error in (no error)"=w257, "Settings"=w254, "Comm Config In"=w255) -> ("error out"=w263:errorcluster)  [unwired: 2 in, 4 out]
                    n139 = call "Time Delay9"("error in (no error)"=w263, "Delay Time (s)"=w253) -> ("error out"=w262:errorcluster)  [unwired: 9 in]
                    n140 = global write "cRIO_ZNB_AMI_GLOBALES.vi" "Remote SET Z"(FALSE ("Remote SET X")) -> ()
                    n141 = local write "Remote SET Z"(FALSE ("Remote SET X")) -> ()
                    n142 = local write "SET Z"(FALSE ("Remote SET X")) -> ()
                    n143 = call "AMI 430_Hardware_Module_Z AXIS.vi"("Enable"=TRUE, "Command"=AMI_430_Hardware_Module."SET CAMPO", "error in (no error)"=w262, "Settings"=w254, "Comm Config In"=w255) -> ("error out"=w256:errorcluster)  [unwired: 2 in, 4 out]
                  }
                }
                n144 = local write "String"("Cambio parámetros eje Z ..." ("String")) -> ()
              }
            }
          }
          frame "RAMP X" {
            n145 = global read "cRIO_ZNB_AMI_GLOBALES.vi" "Remote RAMP X"() -> (w273:bool)
            n146 = Or(x=w273, y="RAMP X") -> (x .or. y?=w272:bool)
            n147 = case shown="True" w272 {
              tunnel: w278 -> [_ w282]
              tunnel: w277 -> [w279 w286]
              tunnel: [w279 w285] -> w276
              tunnel: w274 -> [_ w284]
              tunnel: "RAMP X" -> [_ w283]
              tunnel: w271 -> [_ _]
              tunnel: w270 -> [_ _]
              tunnel: w268 -> [_ w281]
              frame False {
              }
              frame True {
                # "Si RAMP  X manual o remoto..."
                n148 = case shown="False" w283 {
                  tunnel: w286 -> [w290 w305]
                  tunnel: [w291 w304] -> w285
                  tunnel: w284 -> [w289 w303]
                  tunnel: w281 -> [w288 w300]
                  tunnel: w282 -> [w287 w301]
                  frame False {
                    # "Si RAMP X remoto"
                    n149 = global read "cRIO_ZNB_AMI_GLOBALES.vi" "rampingMode X"() -> (w296:u16)
                    n150 = Bundle By Name(cluster=w287, "rampingMode"=w296) -> (w294:T3)
                    n151 = local write "rampingMode X"(w296) -> ()
                    n152 = local write "Settings X"(w294) -> ()
                    n153 = call "AMI 430_Hardware_Module_X AXIS.vi"("Enable"=TRUE, "Command"=AMI_430_Hardware_Module."SET RAMPING MODE", "error in (no error)"=w290, "Settings"=w294, "Comm Config In"=w288) -> ("error out"=w295:errorcluster)  [unwired: 2 in, 4 out]
                    n154 = global write "cRIO_ZNB_AMI_GLOBALES.vi" "Remote RAMP X"(FALSE ("Remote SET X")) -> ()
                    n155 = local write "Remote RAMP X"(FALSE ("Remote SET X")) -> ()
                    n156 = local write "RAMP X"(FALSE ("Remote SET X")) -> ()
                    n157 = call "Time Delay11"("error in (no error)"=w295, "Delay Time (s)"=w289) -> ("error out"=w291:errorcluster)  [unwired: 9 in]
                  }
                  frame True {
                    # "Si RAMP X manual"
                    n158 = Bundle By Name(cluster=w301, "rampingMode"="rampingMode X") -> (w308:T3)
                    n159 = global write "cRIO_ZNB_AMI_GLOBALES.vi" "rampingMode X"("rampingMode X") -> ()
                    n160 = local write "Settings X"(w308) -> ()
                    n161 = call "AMI 430_Hardware_Module_X AXIS.vi"("Enable"=TRUE, "Command"=AMI_430_Hardware_Module."SET RAMPING MODE", "error in (no error)"=w305, "Settings"=w308, "Comm Config In"=w300) -> ("error out"=w309:errorcluster)  [unwired: 2 in, 4 out]
                    n162 = global write "cRIO_ZNB_AMI_GLOBALES.vi" "Remote RAMP X"(FALSE ("Remote SET X")) -> ()
                    n163 = local write "Remote RAMP X"(FALSE ("Remote SET X")) -> ()
                    n164 = local write "RAMP X"(FALSE ("Remote SET X")) -> ()
                    n165 = call "Time Delay6"("error in (no error)"=w309, "Delay Time (s)"=w303) -> ("error out"=w304:errorcluster)  [unwired: 9 in]
                  }
                }
                n166 = local write "String"("Cambio modo de rampa eje X ..." ("String")) -> ()
              }
            }
          }
          frame "RAMP Y" {
            n167 = global read "cRIO_ZNB_AMI_GLOBALES.vi" "Remote RAMP Y"() -> (w318:bool)
            n168 = Or(x=w318, y="RAMP Y") -> (x .or. y?=w317:bool)
            n169 = case shown="True" w317 {
              tunnel: w323 -> [_ _]
              tunnel: w322 -> [w324 w331]
              tunnel: [w324 w330] -> w321
              tunnel: w319 -> [_ w329]
              tunnel: "RAMP Y" -> [_ w328]
              tunnel: w316 -> [_ _]
              tunnel: w315 -> [_ w326]
              tunnel: w314 -> [_ w327]
              frame False {
              }
              frame True {
                # "Si RAMP  Y manual o remoto..."
                n170 = case shown="False" w328 {
                  tunnel: w331 -> [w335 w350]
                  tunnel: [w336 w349] -> w330
                  tunnel: w329 -> [w334 w348]
                  tunnel: w327 -> [w333 w346]
                  tunnel: w326 -> [w332 w347]
                  frame False {
                    # "Si RAMP Y remoto"
                    n171 = global read "cRIO_ZNB_AMI_GLOBALES.vi" "rampingMode Y"() -> (w341:u16)
                    n172 = Bundle By Name(cluster=w332, "rampingMode"=w341) -> (w339:T3)
                    n173 = local write "rampingMode Y"(w341) -> ()
                    n174 = local write "Settings Y"(w339) -> ()
                    n175 = call "AMI 430_Hardware_Module_Y AXIS.vi"("Enable"=TRUE, "Command"=AMI_430_Hardware_Module."SET RAMPING MODE", "error in (no error)"=w335, "Settings"=w339, "Comm Config In"=w333) -> ("error out"=w340:errorcluster)  [unwired: 2 in, 4 out]
                    n176 = global write "cRIO_ZNB_AMI_GLOBALES.vi" "Remote RAMP Y"(FALSE ("Remote SET X")) -> ()
                    n177 = local write "Remote RAMP Y"(FALSE ("Remote SET X")) -> ()
                    n178 = local write "RAMP Y"(FALSE ("Remote SET X")) -> ()
                    n179 = call "Time Delay16"("error in (no error)"=w340, "Delay Time (s)"=w334) -> ("error out"=w336:errorcluster)  [unwired: 9 in]
                  }
                  frame True {
                    # "Si RAMP Y manual"
                    n180 = Bundle By Name(cluster=w347, "rampingMode"="rampingMode Y") -> (w353:T3)
                    n181 = global write "cRIO_ZNB_AMI_GLOBALES.vi" "rampingMode Y"("rampingMode Y") -> ()
                    n182 = local write "Settings Y"(w353) -> ()
                    n183 = call "AMI 430_Hardware_Module_Y AXIS.vi"("Enable"=TRUE, "Command"=AMI_430_Hardware_Module."SET RAMPING MODE", "error in (no error)"=w350, "Settings"=w353, "Comm Config In"=w346) -> ("error out"=w354:errorcluster)  [unwired: 2 in, 4 out]
                    n184 = global write "cRIO_ZNB_AMI_GLOBALES.vi" "Remote RAMP Y"(FALSE ("Remote SET X")) -> ()
                    n185 = local write "Remote RAMP Y"(FALSE ("Remote SET X")) -> ()
                    n186 = local write "RAMP Y"(FALSE ("Remote SET X")) -> ()
                    n187 = call "Time Delay17"("error in (no error)"=w354, "Delay Time (s)"=w348) -> ("error out"=w349:errorcluster)  [unwired: 9 in]
                  }
                }
                n188 = local write "String"("Cambio modo de rampa eje Y ..." ("String")) -> ()
              }
            }
          }
          frame "RAMP Z" {
            n189 = global read "cRIO_ZNB_AMI_GLOBALES.vi" "Remote RAMP Z"() -> (w363:bool)
            n190 = Or(x=w363, y="RAMP Z") -> (x .or. y?=w362:bool)
            n191 = case shown="True" w362 {
              tunnel: w368 -> [_ _]
              tunnel: w367 -> [w369 w376]
              tunnel: [w369 w375] -> w366
              tunnel: w364 -> [_ w374]
              tunnel: "RAMP Z" -> [_ w373]
              tunnel: w361 -> [_ w371]
              tunnel: w360 -> [_ _]
              tunnel: w358 -> [_ w372]
              frame False {
              }
              frame True {
                # "Si RAMP  Z manual o remoto..."
                n192 = case shown="False" w373 {
                  tunnel: w376 -> [w380 w395]
                  tunnel: [w381 w394] -> w375
                  tunnel: w374 -> [w379 w393]
                  tunnel: w372 -> [w378 w391]
                  tunnel: w371 -> [w377 w392]
                  frame False {
                    # "Si RAMP Z remoto"
                    n193 = global read "cRIO_ZNB_AMI_GLOBALES.vi" "rampingMode Z"() -> (w386:u16)
                    n194 = Bundle By Name(cluster=w377, "rampingMode"=w386) -> (w384:T3)
                    n195 = local write "rampingMode Z"(w386) -> ()
                    n196 = local write "Settings Z"(w384) -> ()
                    n197 = call "AMI 430_Hardware_Module_Z AXIS.vi"("Enable"=TRUE, "Command"=AMI_430_Hardware_Module."SET RAMPING MODE", "error in (no error)"=w380, "Settings"=w384, "Comm Config In"=w378) -> ("error out"=w385:errorcluster)  [unwired: 2 in, 4 out]
                    n198 = global write "cRIO_ZNB_AMI_GLOBALES.vi" "Remote RAMP Z"(FALSE ("Remote SET X")) -> ()
                    n199 = local write "Remote RAMP Z"(FALSE ("Remote SET X")) -> ()
                    n200 = local write "RAMP Z"(FALSE ("Remote SET X")) -> ()
                    n201 = call "Time Delay19"("error in (no error)"=w385, "Delay Time (s)"=w379) -> ("error out"=w381:errorcluster)  [unwired: 9 in]
                  }
                  frame True {
                    # "Si RAMP Z manual"
                    n202 = global write "cRIO_ZNB_AMI_GLOBALES.vi" "rampingMode Z"("rampingMode Z") -> ()
                    n203 = Bundle By Name(cluster=w392, "rampingMode"="rampingMode Z") -> (w398:T3)
                    n204 = local write "Settings Z"(w398) -> ()
                    n205 = call "AMI 430_Hardware_Module_Z AXIS.vi"("Enable"=TRUE, "Command"=AMI_430_Hardware_Module."SET RAMPING MODE", "error in (no error)"=w395, "Settings"=w398, "Comm Config In"=w391) -> ("error out"=w399:errorcluster)  [unwired: 2 in, 4 out]
                    n206 = global write "cRIO_ZNB_AMI_GLOBALES.vi" "Remote RAMP Z"(FALSE ("Remote SET X")) -> ()
                    n207 = local write "Remote RAMP Z"(FALSE ("Remote SET X")) -> ()
                    n208 = local write "RAMP Z"(FALSE ("Remote SET X")) -> ()
                    n209 = call "Time Delay20"("error in (no error)"=w399, "Delay Time (s)"=w393) -> ("error out"=w394:errorcluster)  [unwired: 9 in]
                  }
                }
                n210 = local write "String"("Cambio modo de rampa eje Z ..." ("String")) -> ()
              }
            }
          }
          frame "DESIMANAR X" {
            n211 = global read "cRIO_ZNB_AMI_GLOBALES.vi" "Remote DEMAG X"() -> (w408:bool)
            n212 = Or(x=w408, y="Demag X") -> (x .or. y?=w407:bool)
            n213 = case shown="True" w407 {
              tunnel: w413 -> [_ w417]
              tunnel: w412 -> [w414 w421]
              tunnel: [w414 w420] -> w411
              tunnel: w409 -> [_ w419]
              tunnel: "Demag X" -> [_ w418]
              tunnel: w406 -> [_ _]
              tunnel: w405 -> [_ _]
              tunnel: w404 -> [_ w416]
              frame False {
              }
              frame True {
                # "Si DEMAG  X manual o remoto..."
                n214 = case shown="True" w418 {
                  tunnel: w421 -> [w422 w435]
                  tunnel: [w422 w439] -> w420
                  tunnel: w419 -> [_ w425]
                  tunnel: w416 -> [_ w433]
                  tunnel: w417 -> [_ w438]
                  frame False {
                    # "Si RAMP X remoto"
                  }
                  frame True {
                    w437 = u16 0 items=["RAMP", "PAUSE", "MANUAL UP", "MANUAL DOWN", "ZERO"] ("rampingMode X 2")
                    # "Si RAMP X manual"
                    n215 = call "AMI_Desimana X axis.vi"("error in (no error)"=w435) -> ("error out"=w434:errorcluster, "resulting string X"=w436:string)  [unwired: 7 in]
                    n216 = call "AMI_Parse_Desimanar_X.vi"("error in (no error)"=w434, "String"=w436) -> ("error out"=w430:errorcluster, "X Wait secs"=w424:dbl, "X Rate"=w428:dbl, "X Steps"=w429:i32)  [unwired: 6 in]
                    n217 = Bundle By Name(cluster=w438, "rampingMode"=w437) -> (w432:T3)
                    n218 = global write "cRIO_ZNB_AMI_GLOBALES.vi" "rampingMode X"(w437) -> ()
                    n219 = local write "rampingMode X"(w437) -> ()
                    n220 = global read "cRIO_ZNB_AMI_GLOBALES.vi" "X field (T)"() -> (w427:dbl)
                    n221 = call "Demag_fields.vi"("error in (no error)"=w430, "Steps"=w429, "Field (T)"=w427) -> ("error out"=w431:errorcluster, "Fields"=w426:dbl[])  [unwired: 7 in]
                    n222 = local write "Settings X"(w432) -> ()
                    n223 = for {
                      tunnel: w425 -> [w447]
                      tunnel: w433 -> [w440]
                      tunnel: w432 -> [w451]
                      shift-right: [w445] -> w439
                      shift-left: w431 -> [w449]
                      tunnel: w428 -> [w442]
                      tunnel: w426 -> [w441] mode=indexing
                      tunnel: w424 -> [w444]
                      tunnel: [FALSE ("Remote SET X")] -> w423
                      n224 = Bundle By Name(cluster=w451, "targetField"=w441, "rampRate"=w442) -> (w450:T3)
                      n225 = global write "cRIO_ZNB_AMI_GLOBALES.vi" "Rate X(T/min)"(w442) -> ()
                      n226 = local write "Rate X(T/min)"(w442) -> ()
                      n227 = global write "cRIO_ZNB_AMI_GLOBALES.vi" "Target X(T)"(w441) -> ()
                      n228 = local write "Target X(T)"(w441) -> ()
                      n229 = local write "Settings X"(w450) -> ()
                      n230 = call "AMI 430_Hardware_Module_X AXIS.vi"("Enable"=TRUE, "Command"=AMI_430_Hardware_Module."SET  RAMPA", "error in (no error)"=w449, "Settings"=w450, "Comm Config In"=w440) -> ("error out"=w458:errorcluster)  [unwired: 2 in, 4 out]
                      n231 = call "Time Delay7"("error in (no error)"=w458, "Delay Time (s)"=w447) -> ("error out"=w459:errorcluster)  [unwired: 9 in]
                      n232 = call "AMI 430_Hardware_Module_X AXIS.vi"("Enable"=TRUE, "Command"=AMI_430_Hardware_Module."SET CAMPO", "error in (no error)"=w459, "Settings"=w450, "Comm Config In"=w440) -> ("error out"=w453:errorcluster)  [unwired: 2 in, 4 out]
                      n233 = call "Time Delay12"("error in (no error)"=w453, "Delay Time (s)"=w447) -> ("error out"=w452:errorcluster)  [unwired: 9 in]
                      n234 = call "AMI 430_Hardware_Module_X AXIS.vi"("Enable"=TRUE, "Command"=AMI_430_Hardware_Module."SET RAMPING MODE", "error in (no error)"=w452, "Settings"=w450, "Comm Config In"=w440) -> ("error out"=w462:errorcluster)  [unwired: 2 in, 4 out]
                      n235 = call "Time Delay10"("error in (no error)"=w462, "Delay Time (s)"=w447) -> ("error out"=w448:errorcluster)  [unwired: 9 in]
                      n236 = while {
                        shift-right: [w468] -> w446
                        shift-left: w448 -> [w470]
                        tunnel: w447 -> [w467]
                        tunnel: w440 -> [w463]
                        stop <- w465 stop-if-true
                        w473 = T2 1 items=["Unknown", "RAMPING to target field/current", "HOLDING at the target field/current", "PAUSED", "Ramping in MANUAL UP mode", "Ramping in MANUAL DOWN mode", "ZEROING CURRENT (in progress)", "Quench detected", "At ZERO current", "Heating persistent switch", "Cooling persistent switch", "External Rampdown active"] ("y")
                        n237 = property on="Refresh" class="Bool (strict)"(error in=w470, "Value"=TRUE ("Refresh")) -> (error out=w475:errorcluster)  [unwired: 1 in, 1 out]
                        n238 = call "AMI 430_Hardware_Module_X AXIS.vi"("Enable"=TRUE, "Command"=AMI_430_Hardware_Module."READ CAMPO", "error in (no error)"=w475, "Comm Config In"=w463) -> ("error out"=w482:errorcluster, "magneticField"=w485:dbl)  [unwired: 3 in, 3 out]
                        n239 = call "AMI 430_Hardware_Module_X AXIS.vi"("Enable"=TRUE, "Command"=AMI_430_Hardware_Module."STATUS", "error in (no error)"=w482, "Comm Config In"=w463) -> ("error out"=w474:errorcluster, "state"=w472:T2)  [unwired: 3 in, 3 out]
                        n240 = global read "cRIO_ZNB_AMI_GLOBALES.vi" "Z field (T)"() -> (w483:dbl)
                        n241 = global read "cRIO_ZNB_AMI_GLOBALES.vi" "Y field (T)"() -> (w484:dbl)
                        n242 = global write "cRIO_ZNB_AMI_GLOBALES.vi" "X field (T)"(w485) -> ()
                        n243 = local write "X field (T)"(w485) -> ()
                        n244 = global write "cRIO_ZNB_AMI_GLOBALES.vi" "X state"(w472) -> ()
                        n245 = local write "X state"(w472) -> ()
                        n246 = property on="Refresh" class="Bool (strict)"(error in=w474, "Value"=FALSE ("Refresh")) -> (error out=w469:errorcluster)  [unwired: 1 in, 1 out]
                        n247 = Equal?(x=w472, y=w473) -> (x = y?=w471:bool)
                        n248 = Bundle("Z field (T)"=w483, "Y field (T)"=w484, "magneticField"=w485) -> (w486:T7)  [unwired: 1 in]
                        n249 = local write "X ramping"(w471) -> ()
                        n250 = global write "cRIO_ZNB_AMI_GLOBALES.vi" "X ramping"(w471) -> ()
                        n251 = local write "Waveform Chart"(w486) -> ()
                        n252 = call "Time Delay13"("error in (no error)"=w469, "Delay Time (s)"=w467) -> ("error out"=w468:errorcluster)  [unwired: 9 in]
                        n253 = Not(x=w471) -> (.not. x?=w466:bool)
                        n254 = Or(x=w466, y=FALSE ("Refresh")) -> (x .or. y?=w465:bool)
                      }
                      n255 = call "Time Delay14"("error in (no error)"=w446, "Delay Time (s)"=w444) -> ("error out"=w445:errorcluster)  [unwired: 9 in]
                    }
                    n256 = global write "cRIO_ZNB_AMI_GLOBALES.vi" "Remote DEMAG X"(w423) -> ()
                    n257 = local write "Remote DEMAG X"(w423) -> ()
                    n258 = local write "Demag X"(w423) -> ()
                  }
                }
                n259 = local write "String"("Desmagnetizando eje X ... ESPERE..." ("String")) -> ()
              }
            }
          }
          frame "DESIMANAR Y" {
            n260 = global read "cRIO_ZNB_AMI_GLOBALES.vi" "Remote DEMAG Y"() -> (w492:bool)
            n261 = Or(x=w492, y="Demag Y") -> (x .or. y?=w491:bool)
            n262 = case shown="True" w491 {
              tunnel: w497 -> [_ w502]
              tunnel: w496 -> [w498 w506]
              tunnel: [w498 w505] -> w495
              tunnel: w493 -> [_ w504]
              tunnel: "Demag Y" -> [_ w503]
              tunnel: w490 -> [_ _]
              tunnel: w489 -> [_ w499]
              tunnel: w487 -> [_ w501]
              frame False {
              }
              frame True {
                # "Si DEMAG  Y manual o remoto..."
                n263 = case shown="True" w503 {
                  tunnel: w506 -> [w507 w521]
                  tunnel: [w507 w524] -> w505
                  tunnel: w504 -> [_ w511]
                  tunnel: w501 -> [_ w519]
                  tunnel: w502 -> [_ _]
                  tunnel: w499 -> [_ w508]
                  frame False {
                    # "Si RAMP Y remoto"
                  }
                  frame True {
                    w523 = u16 0 items=["RAMP", "PAUSE", "MANUAL UP", "MANUAL DOWN", "ZERO"] ("rampingMode X 2")
                    # "Si RAMP Y manual"
                    n264 = call "AMI_Desimana Y axis.vi"("error in (no error)"=w521) -> ("error out"=w520:errorcluster, "resulting string Y"=w522:string)  [unwired: 7 in]
                    n265 = call "AMI_Parse_Desimanar_Y.vi"("error in (no error)"=w520, "String"=w522) -> ("error out"=w516:errorcluster, "Y Wait secs"=w510:i32, "Y Rate"=w514:dbl, "Y Steps"=w515:i32)  [unwired: 6 in]
                    n266 = Bundle By Name(cluster=w508, "rampingMode"=w523) -> (w518:T3)
                    n267 = global write "cRIO_ZNB_AMI_GLOBALES.vi" "rampingMode Y"(w523) -> ()
                    n268 = local write "rampingMode Y"(w523) -> ()
                    n269 = global read "cRIO_ZNB_AMI_GLOBALES.vi" "Y field (T)"() -> (w513:dbl)
                    n270 = call "Demag_fields.vi"("error in (no error)"=w516, "Steps"=w515, "Field (T)"=w513) -> ("error out"=w517:errorcluster, "Fields"=w512:dbl[])  [unwired: 7 in]
                    n271 = local write "Settings Y"(w518) -> ()
                    n272 = for {
                      tunnel: w511 -> [w532]
                      tunnel: w519 -> [w525]
                      tunnel: w518 -> [w536]
                      shift-right: [w530] -> w524
                      shift-left: w517 -> [w534]
                      tunnel: w514 -> [w527]
                      tunnel: w512 -> [w526] mode=indexing
                      tunnel: w510 -> [w529]
                      tunnel: [FALSE ("Remote SET X")] -> w509
                      n273 = Bundle By Name(cluster=w536, "targetField"=w526, "rampRate"=w527) -> (w535:T3)
                      n274 = global write "cRIO_ZNB_AMI_GLOBALES.vi" "Rate Y(T/min)"(w527) -> ()
                      n275 = local write "Rate Y(T/min)"(w527) -> ()
                      n276 = global write "cRIO_ZNB_AMI_GLOBALES.vi" "Target Y(T)"(w526) -> ()
                      n277 = local write "Target Y(T)"(w526) -> ()
                      n278 = local write "Settings Y"(w535) -> ()
                      n279 = call "AMI 430_Hardware_Module_Y AXIS.vi"("Enable"=TRUE, "Command"=AMI_430_Hardware_Module."SET  RAMPA", "error in (no error)"=w534, "Settings"=w535, "Comm Config In"=w525) -> ("error out"=w543:errorcluster)  [unwired: 2 in, 4 out]
                      n280 = call "Time Delay21"("error in (no error)"=w543, "Delay Time (s)"=w532) -> ("error out"=w544:errorcluster)  [unwired: 9 in]
                      n281 = call "AMI 430_Hardware_Module_Y AXIS.vi"("Enable"=TRUE, "Command"=AMI_430_Hardware_Module."SET CAMPO", "error in (no error)"=w544, "Settings"=w535, "Comm Config In"=w525) -> ("error out"=w538:errorcluster)  [unwired: 2 in, 4 out]
                      n282 = call "Time Delay22"("error in (no error)"=w538, "Delay Time (s)"=w532) -> ("error out"=w537:errorcluster)  [unwired: 9 in]
                      n283 = call "AMI 430_Hardware_Module_Y AXIS.vi"("Enable"=TRUE, "Command"=AMI_430_Hardware_Module."SET RAMPING MODE", "error in (no error)"=w537, "Settings"=w535, "Comm Config In"=w525) -> ("error out"=w547:errorcluster)  [unwired: 2 in, 4 out]
                      n284 = call "Time Delay18"("error in (no error)"=w547, "Delay Time (s)"=w532) -> ("error out"=w533:errorcluster)  [unwired: 9 in]
                      n285 = while {
                        shift-right: [w555] -> w531
                        shift-left: w533 -> [w557]
                        tunnel: w532 -> [w554]
                        tunnel: w525 -> [w548]
                        stop <- w552 stop-if-true
                        w560 = T2 1 items=["Unknown", "RAMPING to target field/current", "HOLDING at the target field/current", "PAUSED", "Ramping in MANUAL UP mode", "Ramping in MANUAL DOWN mode", "ZEROING CURRENT (in progress)", "Quench detected", "At ZERO current", "Heating persistent switch", "Cooling persistent switch", "External Rampdown active"] ("y")
                        n286 = property on="Refresh" class="Bool (strict)"(error in=w557, "Value"=TRUE ("Refresh")) -> (error out=w562:errorcluster)  [unwired: 1 in, 1 out]
                        n287 = call "AMI 430_Hardware_Module_Y AXIS.vi"("Enable"=TRUE, "Command"=AMI_430_Hardware_Module."READ CAMPO", "error in (no error)"=w562, "Comm Config In"=w548) -> ("error out"=w569:errorcluster, "magneticField"=w549:dbl)  [unwired: 3 in, 3 out]
                        n288 = call "AMI 430_Hardware_Module_Y AXIS.vi"("Enable"=TRUE, "Command"=AMI_430_Hardware_Module."STATUS", "error in (no error)"=w569, "Comm Config In"=w548) -> ("error out"=w561:errorcluster, "state"=w559:T2)  [unwired: 3 in, 3 out]
                        n289 = global read "cRIO_ZNB_AMI_GLOBALES.vi" "Z field (T)"() -> (w570:dbl)
                        n290 = global write "cRIO_ZNB_AMI_GLOBALES.vi" "Y field (T)"(w549) -> ()
                        n291 = global read "cRIO_ZNB_AMI_GLOBALES.vi" "X field (T)"() -> (w550:dbl)
                        n292 = local write "Y field (T)"(w549) -> ()
                        n293 = global write "cRIO_ZNB_AMI_GLOBALES.vi" "Y state"(w559) -> ()
                        n294 = local write "Y state"(w559) -> ()
                        n295 = property on="Refresh" class="Bool (strict)"(error in=w561, "Value"=FALSE ("Refresh")) -> (error out=w556:errorcluster)  [unwired: 1 in, 1 out]
                        n296 = Equal?(x=w559, y=w560) -> (x = y?=w558:bool)
                        n297 = Bundle("Z field (T)"=w570, "magneticField"=w549, "X field (T)"=w550) -> (w571:T8)  [unwired: 1 in]
                        n298 = local write "Y ramping"(w558) -> ()
                        n299 = global write "cRIO_ZNB_AMI_GLOBALES.vi" "Y ramping"(w558) -> ()
                        n300 = local write "Waveform Chart"(w571) -> ()
                        n301 = call "Time Delay23"("error in (no error)"=w556, "Delay Time (s)"=w554) -> ("error out"=w555:errorcluster)  [unwired: 9 in]
                        n302 = Not(x=w558) -> (.not. x?=w553:bool)
                        n303 = Or(x=w553, y=FALSE ("Refresh")) -> (x .or. y?=w552:bool)
                      }
                      n304 = call "Time Delay24"("error in (no error)"=w531, "Delay Time (s)"=w529) -> ("error out"=w530:errorcluster)  [unwired: 9 in]
                    }
                    n305 = global write "cRIO_ZNB_AMI_GLOBALES.vi" "Remote DEMAG Y"(w509) -> ()
                    n306 = local write "Remote DEMAG Y"(w509) -> ()
                    n307 = local write "Demag Y"(w509) -> ()
                  }
                }
                n308 = local write "String"("Desmagnetizando eje Y ... ESPERE..." ("String")) -> ()
              }
            }
          }
          frame "DESIMANAR Z" {
            n309 = global read "cRIO_ZNB_AMI_GLOBALES.vi" "Remote DEMAG Z"() -> (w577:bool)
            n310 = Or(x=w577, y="Demag Z") -> (x .or. y?=w576:bool)
            n311 = case shown="True" w576 {
              tunnel: w582 -> [_ _]
              tunnel: w581 -> [w583 w590]
              tunnel: [w583 w589] -> w580
              tunnel: w578 -> [_ w588]
              tunnel: "Demag Z" -> [_ w587]
              tunnel: w575 -> [_ w584]
              tunnel: w574 -> [_ _]
              tunnel: w572 -> [_ w586]
              frame False {
              }
              frame True {
                # "Si DEMAG  Z manual o remoto..."
                n312 = case shown="True" w587 {
                  tunnel: w590 -> [w591 w605]
                  tunnel: [w591 w608] -> w589
                  tunnel: w588 -> [_ w595]
                  tunnel: w586 -> [_ w603]
                  tunnel: w584 -> [_ w592]
                  frame False {
                    # "Si RAMP Z remoto"
                  }
                  frame True {
                    w607 = u16 0 items=["RAMP", "PAUSE", "MANUAL UP", "MANUAL DOWN", "ZERO"] ("rampingMode X 2")
                    # "Si RAMP Z manual"
                    n313 = call "AMI_Desimana Z axis.vi"("error in (no error)"=w605) -> ("error out"=w604:errorcluster, "resulting string Z"=w606:string)  [unwired: 7 in]
                    n314 = call "AMI_Parse_Desimanar_Z.vi"("error in (no error)"=w604, "String"=w606) -> ("error out"=w600:errorcluster, "Z Wait secs"=w594:i32, "Z Rate"=w598:dbl, "Z Steps"=w599:i32)  [unwired: 6 in]
                    n315 = Bundle By Name(cluster=w592, "rampingMode"=w607) -> (w602:T3)
                    n316 = global write "cRIO_ZNB_AMI_GLOBALES.vi" "rampingMode Z"(w607) -> ()
                    n317 = local write "rampingMode Z"(w607) -> ()
                    n318 = global read "cRIO_ZNB_AMI_GLOBALES.vi" "Z field (T)"() -> (w597:dbl)
                    n319 = call "Demag_fields.vi"("error in (no error)"=w600, "Steps"=w599, "Field (T)"=w597) -> ("error out"=w601:errorcluster, "Fields"=w596:dbl[])  [unwired: 7 in]
                    n320 = local write "Settings Z"(w602) -> ()
                    n321 = for {
                      tunnel: w595 -> [w616]
                      tunnel: w603 -> [w609]
                      tunnel: w602 -> [w620]
                      shift-right: [w614] -> w608
                      shift-left: w601 -> [w618]
                      tunnel: w598 -> [w611]
                      tunnel: w596 -> [w610] mode=indexing
                      tunnel: w594 -> [w613]
                      tunnel: [FALSE ("Remote SET X")] -> w593
                      n322 = Bundle By Name(cluster=w620, "targetField"=w610, "rampRate"=w611) -> (w619:T3)
                      n323 = global write "cRIO_ZNB_AMI_GLOBALES.vi" "Rate Z(T/min)"(w611) -> ()
                      n324 = local write "Rate Z(T/min)"(w611) -> ()
                      n325 = global write "cRIO_ZNB_AMI_GLOBALES.vi" "Target Z(T)"(w610) -> ()
                      n326 = local write "Target Z(T)"(w610) -> ()
                      n327 = local write "Settings Z"(w619) -> ()
                      n328 = call "AMI 430_Hardware_Module_Z AXIS.vi"("Enable"=TRUE, "Command"=AMI_430_Hardware_Module."SET  RAMPA", "error in (no error)"=w618, "Settings"=w619, "Comm Config In"=w609) -> ("error out"=w627:errorcluster)  [unwired: 2 in, 4 out]
                      n329 = call "Time Delay27"("error in (no error)"=w627, "Delay Time (s)"=w616) -> ("error out"=w628:errorcluster)  [unwired: 9 in]
                      n330 = call "AMI 430_Hardware_Module_Z AXIS.vi"("Enable"=TRUE, "Command"=AMI_430_Hardware_Module."SET CAMPO", "error in (no error)"=w628, "Settings"=w619, "Comm Config In"=w609) -> ("error out"=w622:errorcluster)  [unwired: 2 in, 4 out]
                      n331 = call "Time Delay28"("error in (no error)"=w622, "Delay Time (s)"=w616) -> ("error out"=w621:errorcluster)  [unwired: 9 in]
                      n332 = call "AMI 430_Hardware_Module_Z AXIS.vi"("Enable"=TRUE, "Command"=AMI_430_Hardware_Module."SET RAMPING MODE", "error in (no error)"=w621, "Settings"=w619, "Comm Config In"=w609) -> ("error out"=w631:errorcluster)  [unwired: 2 in, 4 out]
                      n333 = call "Time Delay26"("error in (no error)"=w631, "Delay Time (s)"=w616) -> ("error out"=w617:errorcluster)  [unwired: 9 in]
                      n334 = while {
                        shift-right: [w639] -> w615
                        shift-left: w617 -> [w641]
                        tunnel: w616 -> [w638]
                        tunnel: w609 -> [w632]
                        stop <- w636 stop-if-true
                        w644 = T2 1 items=["Unknown", "RAMPING to target field/current", "HOLDING at the target field/current", "PAUSED", "Ramping in MANUAL UP mode", "Ramping in MANUAL DOWN mode", "ZEROING CURRENT (in progress)", "Quench detected", "At ZERO current", "Heating persistent switch", "Cooling persistent switch", "External Rampdown active"] ("y")
                        n335 = property on="Refresh" class="Bool (strict)"(error in=w641, "Value"=TRUE ("Refresh")) -> (error out=w646:errorcluster)  [unwired: 1 in, 1 out]
                        n336 = call "AMI 430_Hardware_Module_Z AXIS.vi"("Enable"=TRUE, "Command"=AMI_430_Hardware_Module."READ CAMPO", "error in (no error)"=w646, "Comm Config In"=w632) -> ("error out"=w653:errorcluster, "magneticField"=w634:dbl)  [unwired: 3 in, 3 out]
                        n337 = call "AMI 430_Hardware_Module_Z AXIS.vi"("Enable"=TRUE, "Command"=AMI_430_Hardware_Module."STATUS", "error in (no error)"=w653, "Comm Config In"=w632) -> ("error out"=w645:errorcluster, "state"=w643:T2)  [unwired: 3 in, 3 out]
                        n338 = global write "cRIO_ZNB_AMI_GLOBALES.vi" "Z field (T)"(w634) -> ()
                        n339 = global read "cRIO_ZNB_AMI_GLOBALES.vi" "Y field (T)"() -> (w654:dbl)
                        n340 = global read "cRIO_ZNB_AMI_GLOBALES.vi" "X field (T)"() -> (w633:dbl)
                        n341 = local write "Z field (T)"(w634) -> ()
                        n342 = global write "cRIO_ZNB_AMI_GLOBALES.vi" "Z state"(w643) -> ()
                        n343 = local write "Z state"(w643) -> ()
                        n344 = property on="Refresh" class="Bool (strict)"(error in=w645, "Value"=FALSE ("Refresh")) -> (error out=w640:errorcluster)  [unwired: 1 in, 1 out]
                        n345 = Equal?(x=w643, y=w644) -> (x = y?=w642:bool)
                        n346 = Bundle("magneticField"=w634, "Y field (T)"=w654, "X field (T)"=w633) -> (w655:T9)  [unwired: 1 in]
                        n347 = local write "Z ramping"(w642) -> ()
                        n348 = global write "cRIO_ZNB_AMI_GLOBALES.vi" "Z ramping"(w642) -> ()
                        n349 = local write "Waveform Chart"(w655) -> ()
                        n350 = call "Time Delay29"("error in (no error)"=w640, "Delay Time (s)"=w638) -> ("error out"=w639:errorcluster)  [unwired: 9 in]
                        n351 = Not(x=w642) -> (.not. x?=w637:bool)
                        n352 = Or(x=w637, y=FALSE ("Refresh")) -> (x .or. y?=w636:bool)
                      }
                      n353 = call "Time Delay30"("error in (no error)"=w615, "Delay Time (s)"=w613) -> ("error out"=w614:errorcluster)  [unwired: 9 in]
                    }
                    n354 = global write "cRIO_ZNB_AMI_GLOBALES.vi" "Remote DEMAG Z"(w593) -> ()
                    n355 = local write "Remote DEMAG Z"(w593) -> ()
                    n356 = local write "Demag Z"(w593) -> ()
                  }
                }
                n357 = local write "String"("Desmagnetizando eje Z ... ESPERE..." ("String")) -> ()
              }
            }
          }
        }
        "Command" <- w54
        n358 = global read "cRIO_ZNB_AMI_GLOBALES.vi" "stopMagneticField"() -> (w67:bool)
        n359 = Unbundle By Name(w62) -> ("status"=→"ERROR":bool)
        n360 = call <vilib>:"Clear Errors.vi"("error in (no error)"=w62) -> ("error out"=w65:errorcluster)  [unwired: 5 in, 1 out]
        n361 = control-ref of="This VI"() -> (w68:refnum<vi>)
        n362 = Or(x="stop", y=w67) -> (x .or. y?=w72:bool)
        "Ciclo" <- w64
      }
      "Error Out" <- w50
      n363 = global write "cRIO_ZNB_AMI_GLOBALES.vi" "stopMagneticField"(w51) -> ()
      n364 = invoke class="VI" method="FP.Close"(reference=w52) -> ()  [unwired: 2 in, 3 out]
      "Remote SET Y" <- w11
      "Remote RAMP X" <- w14
      "Remote SET X" <- w13
      "Remote RAMP Z" <- w16
      "Remote SET Z" <- w12
      "Remote RAMP Y" <- w15
      "Remote DEMAG Y" <- w7
      "Remote DEMAG X" <- w6
      "Remote DEMAG Z" <- w5
    }
  }
  "String" <- w1
